vi "FGV Read-write settings-to-Miyachi.vi"(9 "VISA resource name":refnum<visa-resource-name>="COM1", 10 "Soldadora":i32=1, 11 "Linea":i32=1) -> (3 "STATUS":u32(colorbox))   [LabVIEW 2014]
uses:
  control/FGV Variables State machine.ctl
  control/FGV Machine states.ctl
  control/FGV Comandos.ctl
  control/FGV Escribir datos a miyachi-booleano.ctl
  control/FGV Lectura.ctl
  control/FGV botones Read-Write.ctl
  control/FGV Select case.ctl
panel:
  out "current time":timestamp
  in  "min/seg 2":u16(ring) items=["seg", "min"]
  in  "Time update":i32=5
  in  "Exit":bool
  in  "Botones r-w":T1
  out "CURRENT #2":dbl
  out "CURRENT #1":dbl
  out "VOLTLOW2":dbl
  out "VOLTHIW2":dbl
  out "VOLTLOW1":dbl
  out "VOLTHIW1":dbl
  out "Weld mode":i32
  out "Start value":i32
  out "sold1_error_fromLV":bool
  out "sold1_warning_fromLV":bool
  out "error out":errorcluster
  in  "Variables R-W":T2={"Máquina"=0.0, "Error STA"=0.0, "Contador de veces"=0.0, "Timeout"=0.0, "Tiempo"=0.0, "State"=enum."Start", "error in (no error)"={"status"=FALSE, "code"=0, "source"=""}, "error out"={"status"=FALSE, "code"=0, "source"=""}, "Msg Error"="", "Leer comando"="", "up sol"=0.0, "VISA resource name"="", "Comando a recibir"=enum."ACK", "Comando que sigue"=enum."Ninguno", "Modo escritura"=enum."No", "Modo lectura"=enum."No", "Estado Status"=enum."Start", "Botones r-w"={"5"=FALSE, "4"=FALSE, "3"=FALSE, "2"=FALSE, "1"=FALSE}, "stopVI"=FALSE, "Case"=enum."Nada", "Status?"=FALSE, "Soldadora"=0.0}
  in  "error in (no error)":errorcluster
  out "Panel (Local)":bool
  out "PC (Remote)":bool
  out "Local":bool
  out "Remote":bool
  out "FORCE CHANNEL":dbl
  out "Última vez actualizado":string
  out "FORCE":dbl
  out "IMPULSE":dbl
  out "CURRENT #2":string
  out "CURRENT #1":string
  out "%HEAT 2":u32
  out "%HEAT 1":u32
  out "OFF":dbl
  out "HLD":dbl
  out "DN2":dbl
  out "W2":dbl
  out "UP2":dbl
  out "CO":dbl
  out "DN1":dbl
  out "W1":dbl
  out "UP1":dbl
  out "SQZ":dbl
  out "SQD":dbl
  out "Act. SCHE.":dbl
  out "FIRE =":u32
  out "VOLTLOW2":string
  out "VOLTHIW2":string
  out "LO":string
  out "HI":string
  out "HI":dbl
  out "LO":dbl
  out "Weld mode":string
  out "Start value":string
  out "Weld count limit":dbl
  out "Conduction limit #2":dbl
  out "HI":dbl
  out "Low current #2 %":dbl
  out "High current #2 %":dbl
  out "LO":dbl
  out "HI":dbl
  in  "SCHEDULE SET":T8
  in  "MONITOR SET":T9 {"Weld mode" items=["SPOT", "REPEAT", "SUCCESSIVE", "CHAINING"]; "Start value" items=["MAINTAINED", "PULSED", "LATCHED", "SEAM"]}
  in  "SCHEDULE":i32
  in  "SCHEDULE":u32
  out "OK":bool
  # "WELD ON/OFF"
  # "Programming"
  # "CURR(KA)"
  # "COND"
  # "VOLTS"
  # "FORCE(LBS)"
  # "°"
  # "W1"
  # "%"
  # "V"
  # "V"
  # "%"
  # "°"
  # "%"
  # "%"
  # "W2"
  # "V"
  # "V"
  # "Lbs."
  # "VOLTS"
  # "CURR(KA)"
  # "COND"
  # "FORCE(LBS)"
  # "LO"
  # "HI"
  # "HI"
  # "LO"
  # "HI"
  # "LO"
  # "HI"
  # "°"
  # "%"
  # "V"
  # "V"
  # "%"
  # "°"
  # "%"
  # "%"
  # "V"
  # "V"
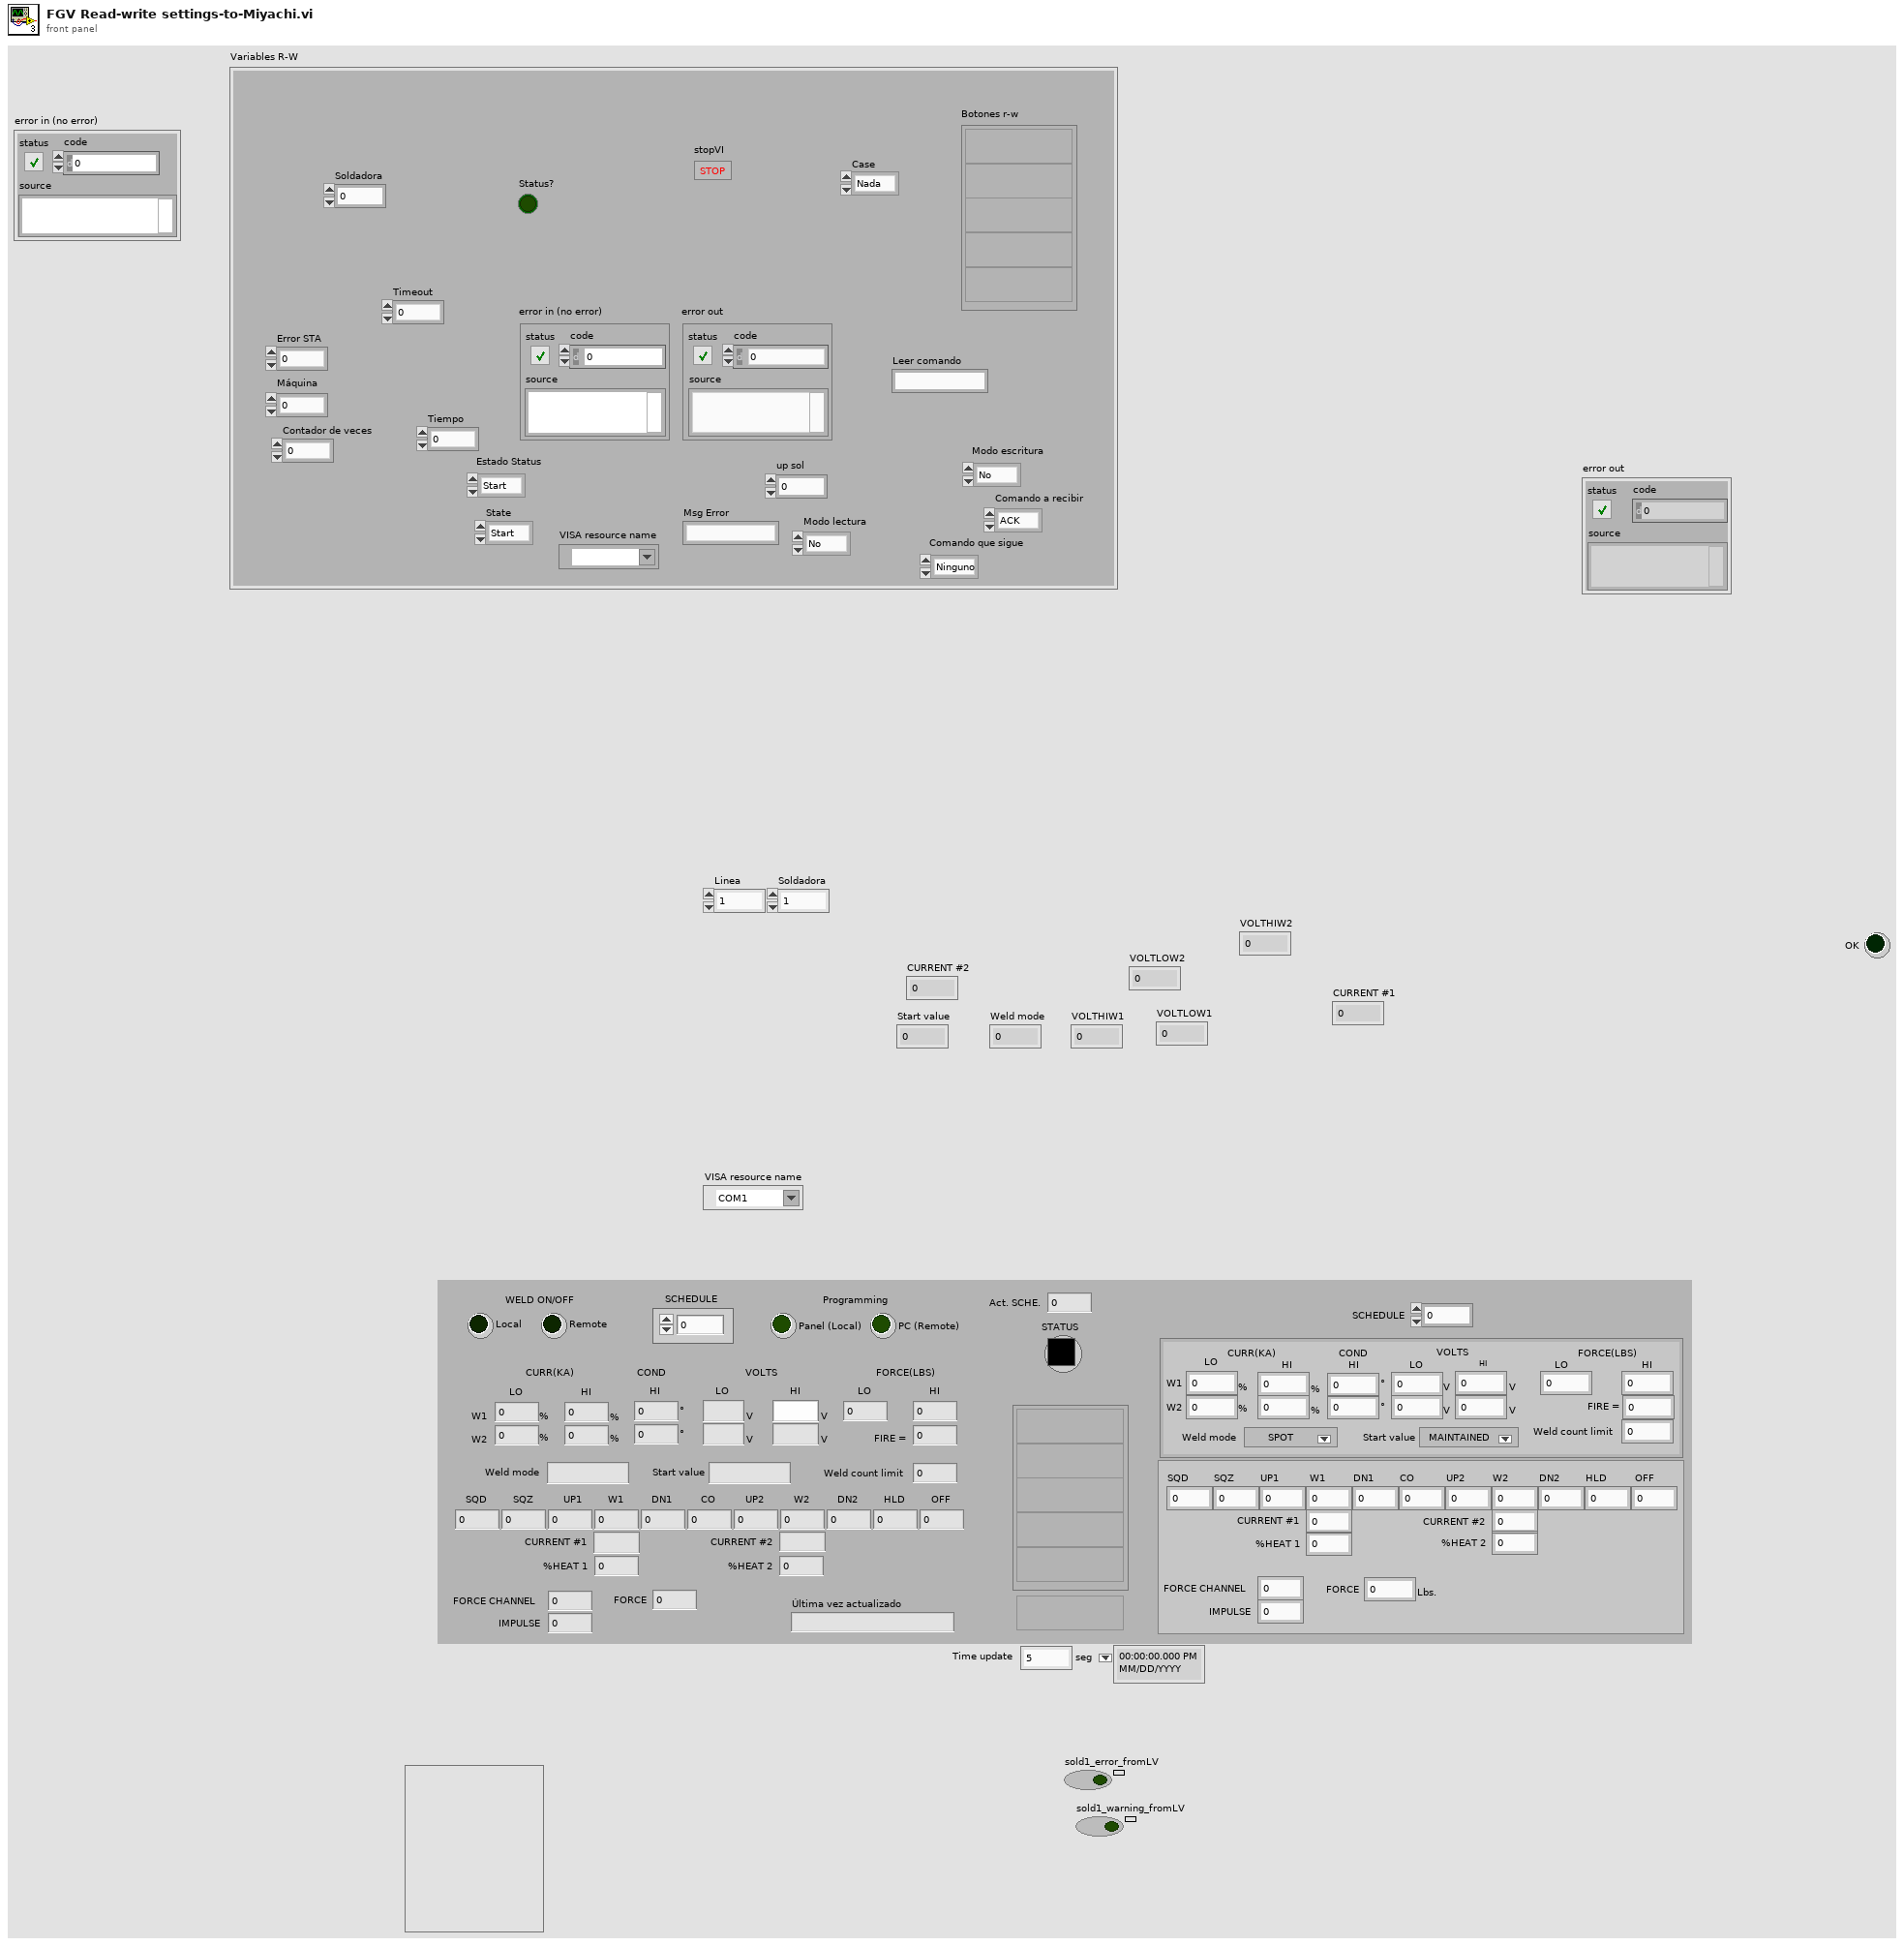
[diagram p1: front panel]
types:
  T1 = typedef "FGV botones Read-Write.ctl" = cluster{"5":bool, "4":bool, "3":bool, "2":bool, "1":bool}
  T2 = typedef "FGV Variables State machine.ctl" = cluster{"Máquina":dbl, "Error STA":dbl, "Contador de veces":dbl, "Timeout":dbl, "Tiempo":dbl, "State":T3, "error in (no error)":errorcluster, "error out":errorcluster, "Msg Error":string, "Leer comando":string, "up sol":dbl, "VISA resource name":refnum<visa-resource-name>, "Comando a recibir":T4, "Comando que sigue":T4, "Modo escritura":T5, "Modo lectura":T6, "Estado Status":T3, "Botones r-w":T1, "stopVI":bool, "Case":T7, "Status?":bool, "Soldadora":dbl}
  T3 = typedef "FGV Machine states.ctl" = enum16{"Start", "Wait", "Send", "Receive", "Error handler", "Show info", "Do something", "Stop", "Idle"}
  T4 = typedef "FGV Comandos.ctl" = enum16{"Ninguno", "ACK", "Monitor Read", "Schedule Read", "Status Read", "Report Read", "Monitor Set", "Schedule Set", "System Read", "Remote", "Load Read", "Load Set", "Reset"}
  T5 = typedef "FGV Escribir datos a miyachi-booleano.ctl" = enum16{"No", "Si"}
  T6 = typedef "FGV Lectura.ctl" = enum16{"No", "Si"}
  T7 = typedef "FGV Select case.ctl" = enum16{"Nada", "Leer", "Escribir", "Local", "Remote", "Activar Sch."}
  T8 = cluster{"SQD":dbl, "SQZ":dbl, "UP1":dbl, " W1":dbl, "DN1":dbl, "CO":dbl, "UP2":dbl, "W2":dbl, "DN2":dbl, "HLD":dbl, " OFF":dbl, "%HEAT 1":dbl, "%HEAT 2":dbl, "CURRENT #1":dbl, " CURRENT #2":dbl, "IMPULSE":dbl, "FORCE":dbl, "FORCE CHANNEL":dbl}
  T9 = cluster{"HIGH1C":u32, " W1":u32, "HIGH2C":u32, "W2":u32, "ANGLE 1":u32, "ANGLE 2":u32, "Weld count limit":u32, "Start value":u16, "Weld mode":u16, "LOP":dbl, "HIP":dbl, "VOLTHIW1":dbl, "VOLTLOW1":dbl, "VOLTHIW2":dbl, "VOLTLOW2":dbl, "FIRE =":dbl}
  T10 = enum16{"Start", "Wait", "Send", "Receive", "Error handler", "Show info", "Do something", "Stop"}
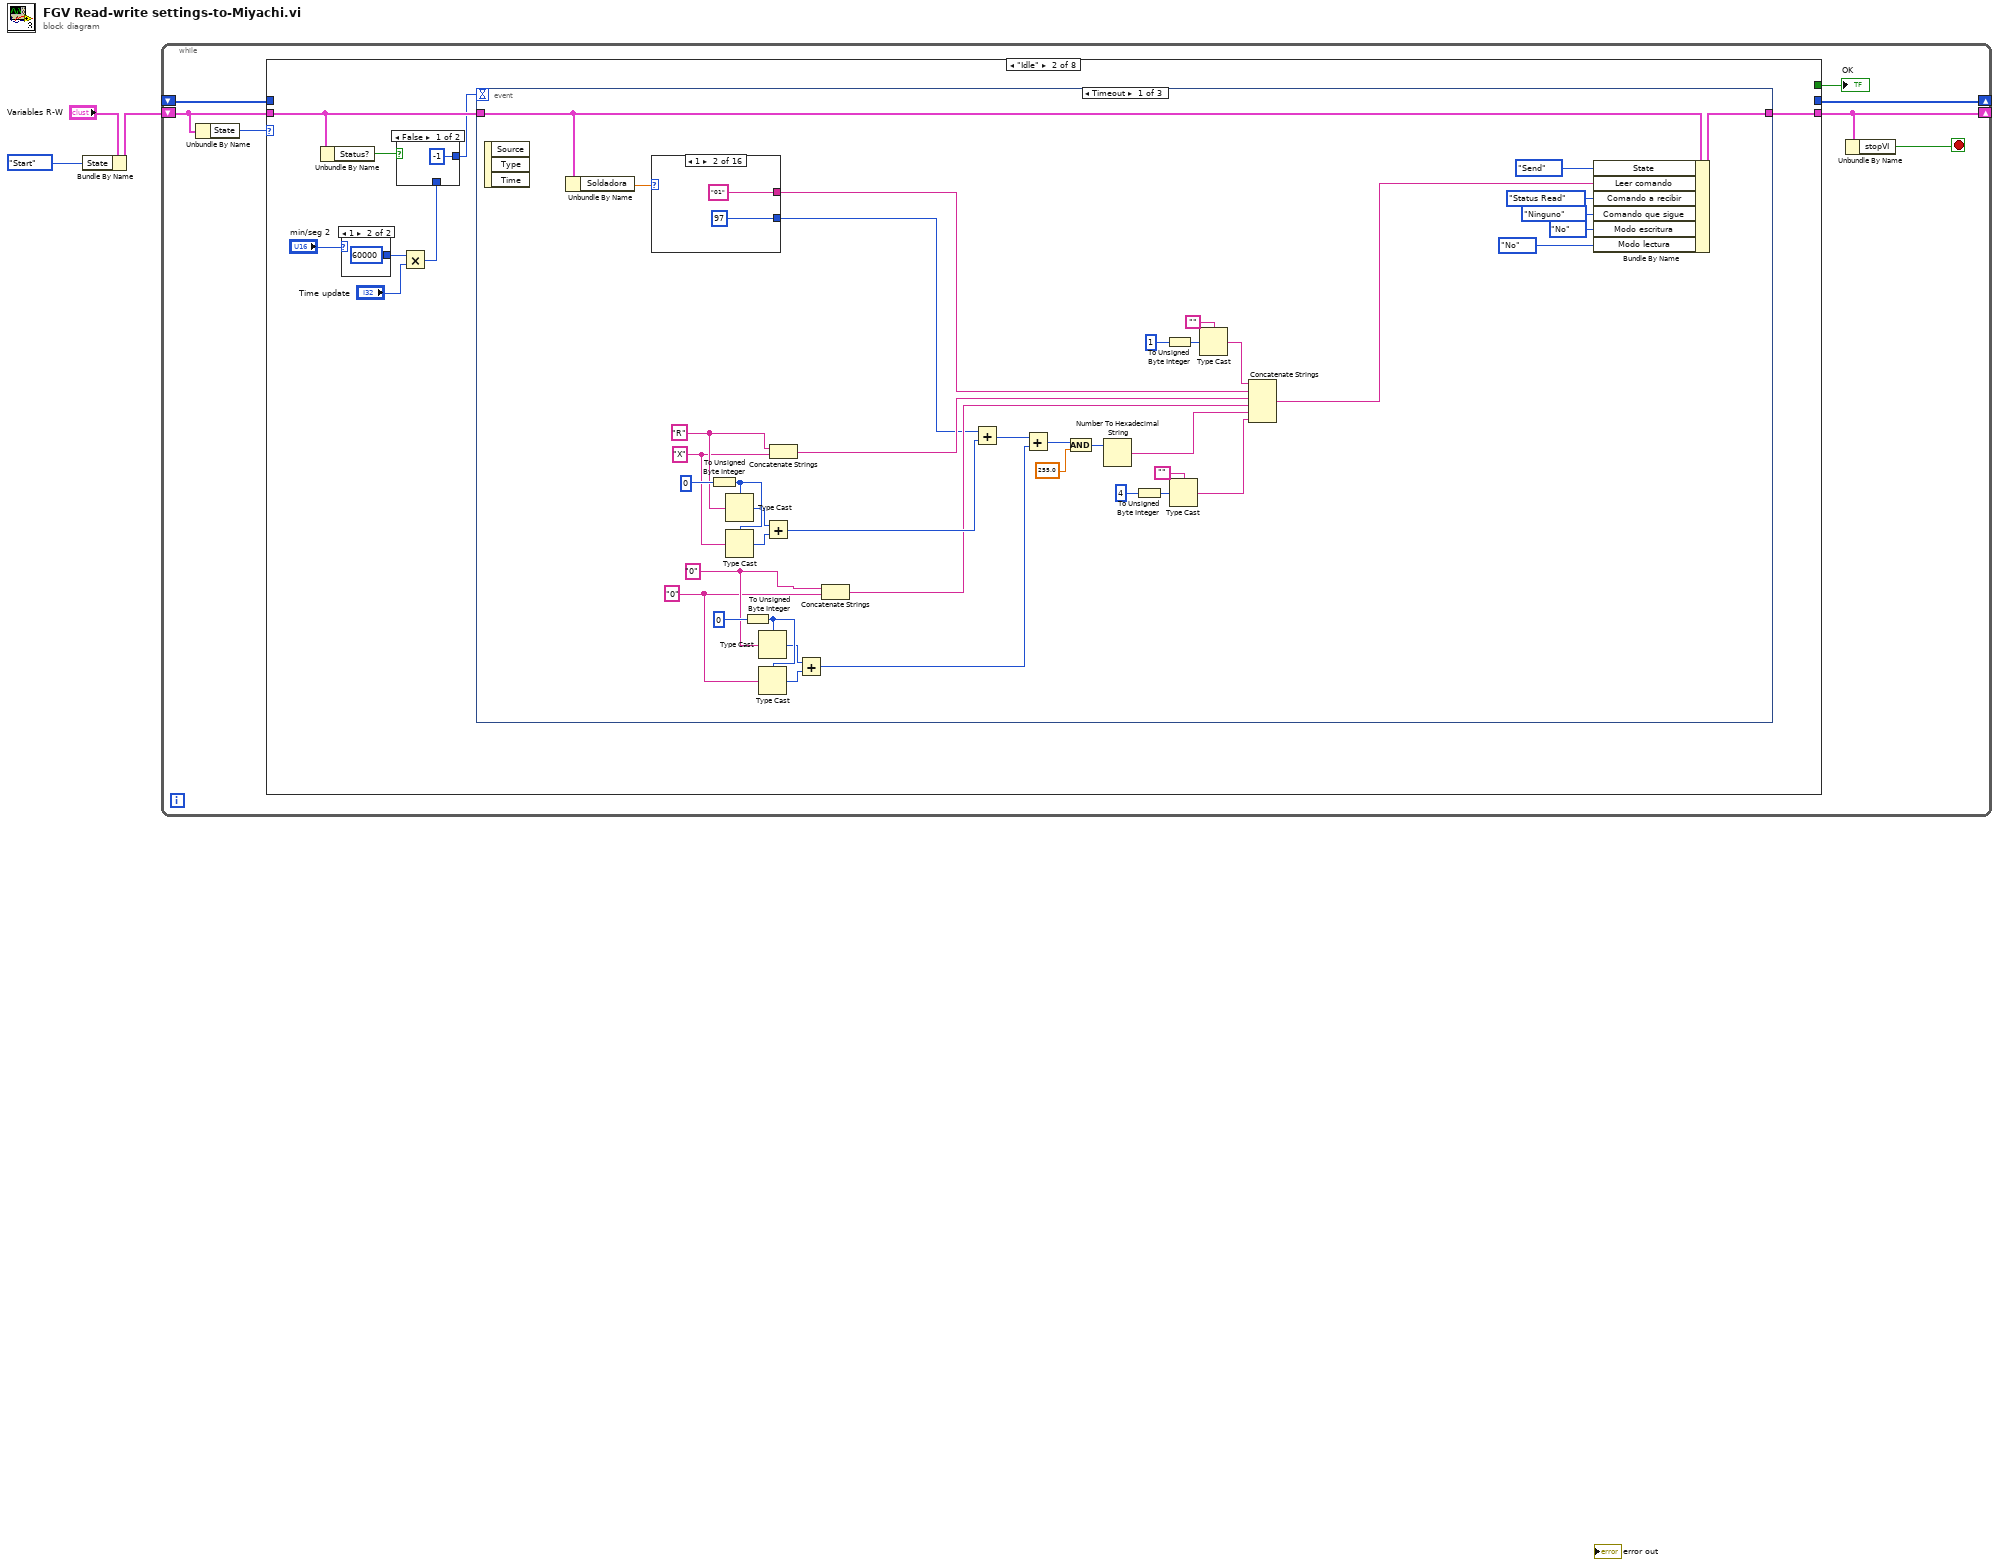
[diagram p0: block diagram]
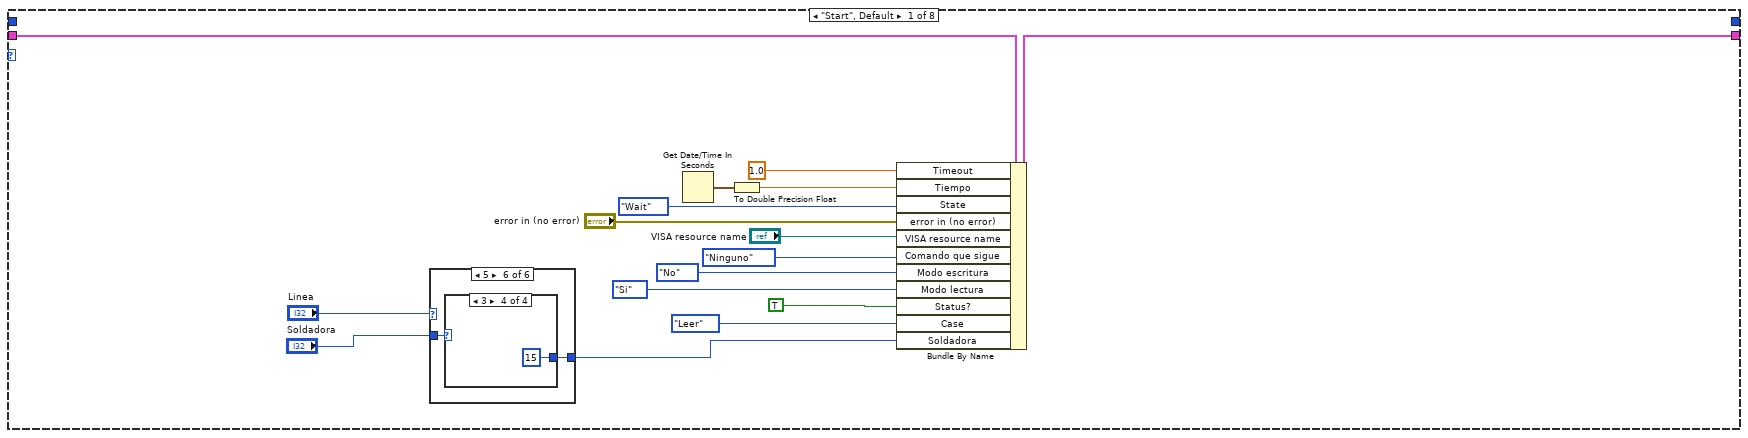
[diagram p2: hidden frame]
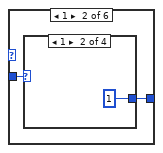
[diagram p4: hidden frame]
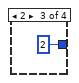
[diagram p6: hidden frame]
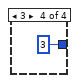
[diagram p7: hidden frame]
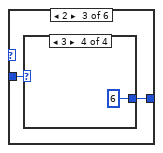
[diagram p8: hidden frame]
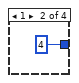
[diagram p10: hidden frame]
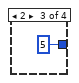
[diagram p11: hidden frame]
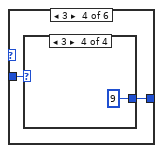
[diagram p12: hidden frame]
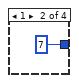
[diagram p14: hidden frame]
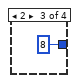
[diagram p15: hidden frame]
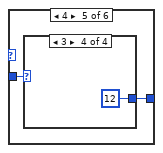
[diagram p16: hidden frame]
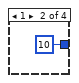
[diagram p18: hidden frame]
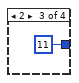
[diagram p19: hidden frame]
diagram:
  n1 = Bundle By Name(cluster="Variables R-W", "State"=FGV_Machine_states."Start" ("Estado R-W")) -> (w1:T2)
  n2 = while {
    shift-right: [w10] -> _
    shift-left: _ -> [w9]
    shift-right: [w5] -> _
    shift-left: w1 -> [w8]
    stop <- w4 stop-if-true
    n3 = Unbundle By Name(w8) -> ("State"=w7:T3)
    n4 = case shown="\"Idle\"" w7 {
      tunnel: [_ _ w192 w523 w537 w597 w747 _] -> w10
      tunnel: w9 -> [_ _ w192 w523 _ w597 w747 _]
      tunnel: [_ _ TRUE FALSE FALSE FALSE FALSE _] -> w6
      tunnel: [w17 w59 w190 w521 w535 w593 w745 w1945] -> w5
      tunnel: w8 -> [w18 w55 w189 w520 w530 w591 w746 w1946]
      frame "Start", Default {
        n5 = case shown="5" "Linea" {
          tunnel: "Soldadora" -> [_ w28 w33 w38 w43 w48]
          tunnel: [_ w27 w32 w37 w42 w47] -> w14
          frame 0, Default {
          }
          frame 1 {
            n6 = case shown="1" w28 {
              tunnel: [_ 1 2 3] -> w27
              frame 0, Default {
              }
              frame 1 {
              }
              frame 2 {
              }
              frame 3 {
              }
            }
          }
          frame 2 {
            n7 = case shown="3" w33 {
              tunnel: [_ 4 5 6] -> w32
              frame 0, Default {
              }
              frame 1 {
              }
              frame 2 {
              }
              frame 3 {
              }
            }
          }
          frame 3 {
            n8 = case shown="3" w38 {
              tunnel: [_ 7 8 9] -> w37
              frame 0, Default {
              }
              frame 1 {
              }
              frame 2 {
              }
              frame 3 {
              }
            }
          }
          frame 4 {
            n9 = case shown="3" w43 {
              tunnel: [_ 10 11 12] -> w42
              frame 0, Default {
              }
              frame 1 {
              }
              frame 2 {
              }
              frame 3 {
              }
            }
          }
          frame 5 {
            n10 = case shown="3" w48 {
              tunnel: [_ 13 14 15] -> w47
              frame 0, Default {
              }
              frame 1 {
              }
              frame 2 {
              }
              frame 3 {
              }
            }
          }
        }
        n11 = Get Date/Time In Seconds() -> (seconds since 1Jan1904=w19:timestamp)
        n12 = To Double Precision Float(number=w19) -> (double precision float=w20:dbl)
        n13 = Bundle By Name(cluster=w18, "Timeout"=1.0, "Tiempo"=w20, "State"=FGV_Machine_states."Wait" ("Estado"), "error in (no error)"="error in (no error)", "VISA resource name"="VISA resource name", "Comando que sigue"=FGV_Comandos."Ninguno" ("Comando en turno"), "Modo escritura"=FGV_Escribir_datos_a_miyachi-booleano."No" ("Escritura?"), "Modo lectura"=FGV_Lectura."Si" ("Lectura"), "Status?"=TRUE, "Case"=FGV_Select_case."Leer", "Soldadora"=w14) -> (w17:T2)
      }
      frame "Idle" {
        n14 = Unbundle By Name(w55) -> ("Status?"=w52:bool)
        n15 = case shown="1" "min/seg 2" {
          tunnel: [1000 60000] -> w58
          frame 0, Default {
          }
          frame 1 {
          }
        }
        n16 = Multiply(x=w58, y="Time update") -> (x*y=w54:i32)
        n17 = case shown="False" w52 {
          tunnel: w54 -> [_ w61]
          tunnel: [-1 w61] -> w53
          frame False {
          }
          frame True {
          }
        }
        n18 = event shown="[0] Timeout" {
          selector: _ -> [_ _ _]
          dyn-events: _ -> [_ _ _]
          timeout: w53 -> [_ _ _]
          tunnel: [w74 w142 w176] -> w59
          tunnel: w55 -> [w71 w136 w177]
          event Timeout {
            w83 = "0" ("string")
            w84 = "0" ("string")
            w95 = "X" ("string")
            w96 = "R" ("string")
            n19 = event-data() -> ()  [unwired: 1 in, 3 out]
            n20 = Unbundle By Name(w71) -> ("Soldadora"=w70:dbl)
            n21 = case shown="1" w70 {
              tunnel: [_ "01" "02" "03" "04" "05" "06" "07" "08" "09" "10" "11" "12" "13" "14" "15"] -> w69
              tunnel: [_ 97 98 99 100 101 102 103 104 105 97 98 99 100 101 102] -> w68
              frame 0, Default {
              }
              frame 1 {
              }
              frame 2 {
              }
              frame 3 {
              }
              frame 4 {
              }
              frame 5 {
              }
              frame 6 {
              }
              frame 7 {
              }
              frame 8 {
              }
              frame 9 {
              }
              frame 10 {
              }
              frame 11 {
              }
              frame 12 {
              }
              frame 13 {
              }
              frame 14 {
              }
              frame 15 {
              }
            }
            n22 = To Unsigned Byte Integer(number=0) -> (unsigned 8bit integer=w99:u8)
            n23 = Type Cast(type=w99, x=w96) -> (*(type *) &x=w98:u8)
            n24 = Type Cast(type=w99, x=w95) -> (*(type *) &x=w97:u8)
            n25 = To Unsigned Byte Integer(number=0) -> (unsigned 8bit integer=w87:u8)
            n26 = Type Cast(type=w87, x=w84) -> (*(type *) &x=w86:u8)
            n27 = Type Cast(type=w87, x=w83) -> (*(type *) &x=w85:u8)
            n28 = Add(x=w98, y=w97) -> (x+y=w91:u8)
            n29 = Concatenate Strings(w96, w95) -> (w79:string)
            n30 = Add(x=w86, y=w85) -> (x+y=w81:u8)
            n31 = Concatenate Strings(w84, w83) -> (w78:string)
            n32 = Add(x=w68, y=w91) -> (x+y=w72:i32)
            n33 = Add(x=w72, y=w81) -> (x+y=w82:i32)
            n34 = And(x=w82, y=255.0) -> (x .and. y?=w89:i32)
            n35 = Number To Hexadecimal String(2:w89) -> (0:w77:string)  [unwired: 1 in]
            n36 = To Unsigned Byte Integer(number=u8 4) -> (unsigned 8bit integer=w94:u8)
            n37 = To Unsigned Byte Integer(number=u8 1) -> (unsigned 8bit integer=w103:u8)
            n38 = Type Cast(type="", x=w94) -> (*(type *) &x=w76:string)
            n39 = Type Cast(type="", x=w103) -> (*(type *) &x=w80:string)
            n40 = Concatenate Strings(w80, w69, w79, w78, w77, w76) -> (w73:string)
            n41 = Bundle By Name(cluster=w71, "State"=FGV_Machine_states."Send" ("Estado R-W"), "Leer comando"=w73, "Comando a recibir"=FGV_Comandos."Status Read", "Comando que sigue"=FGV_Comandos."Ninguno", "Modo escritura"=FGV_Escribir_datos_a_miyachi-booleano."No", "Modo lectura"=FGV_Lectura."No") -> (w74:T2)
          }
          event Value Change {
            n42 = event-data() -> ("CtlRef"=w134:refnum<vi>)  [unwired: 1 in]
            n43 = Cluster To Array(cluster="Botones r-w") -> (array=w148:bool[])
            n44 = for {
              tunnel: w148 -> [w175] mode=indexing
              tunnel: [w174] -> w146
              i -> [w174]
              stop <- w175 stop-if-true
            }
            n45 = property class="Clust"(reference=w134) -> ("Controls[]"=w147:refnum<vi>[])  [unwired: 1 in, 2 out]
            n46 = Index Array(array=w147, index=w146) -> (element=w145:refnum<vi>)
            n47 = Unbundle By Name(w136) -> ("Status?"=w135:bool)
            n48 = property class="Ctl"(reference=w145) -> ("Label.Text"=w144:string)  [unwired: 1 in, 2 out]
            n49 = Decimal String To Number(string=w144) -> (number=w143:i32)  [unwired: 2 in, 1 out]
            n50 = case shown="3" w143 {
              tunnel: [FGV_Machine_states."Idle" ("Estado R-W") FGV_Machine_states."Wait" ("Estado R-W") FGV_Machine_states."Wait" ("Estado R-W") FGV_Machine_states."Wait" ("Estado R-W") FGV_Machine_states."Wait" ("Estado R-W") FGV_Machine_states."Idle" ("Estado R-W")] -> w141
              tunnel: [_ FGV_Lectura."Si" ("Modo lectura") FGV_Lectura."No" ("Modo lectura") FGV_Lectura."No" ("Modo lectura") FGV_Lectura."No" ("Modo lectura") _] -> w140
              tunnel: [_ FGV_Escribir_datos_a_miyachi-booleano."No" ("Modo escritura") FGV_Escribir_datos_a_miyachi-booleano."Si" ("Modo escritura") FGV_Escribir_datos_a_miyachi-booleano."No" ("Modo escritura") FGV_Escribir_datos_a_miyachi-booleano."No" ("Modo escritura") _] -> w139
              tunnel: [_ FGV_Select_case."Leer" ("Case") FGV_Select_case."Escribir" ("Case") FGV_Select_case."Local" ("Case") FGV_Select_case."Remote" ("Case") _] -> w138
              tunnel: [w150 w152 w157 w162 w167 TRUE] -> w137
              tunnel: w135 -> [w150 w152 w157 w162 w167 _]
              frame 0, Default {
              }
              frame 1 {
              }
              frame 2 {
              }
              frame 3 {
              }
              frame 4 {
              }
              frame 5 {
              }
            }
            n51 = Bundle By Name(cluster=w136, "State"=w141, "Modo lectura"=w140, "Modo escritura"=w139, "Case"=w138, "Status?"=w137) -> (w142:T2)
          }
          event "Exit": Value Change {
            n52 = event-data() -> ()  [unwired: 1 in, 6 out]
            n53 = Bundle By Name(cluster=w177, "stopVI"=TRUE) -> (w176:T2)
          }
        }
      }
      frame "Wait" {
        n54 = Unbundle By Name(w189) -> ("Comando que sigue"=w187:T4, "Case"=w180:T7, "Soldadora"=w179:dbl)
        n55 = case shown="\"Escribir\"" w180 {
          tunnel: ["" w220 w297 "\u000101RM01\u000061\u0004" "\u000101RM01\u000162\u0004" "\u000101LS01\u000061\u0004"] -> w188
          tunnel: w187 -> [_ w204 w311 _ _ _]
          tunnel: [w196 w212 w310 FGV_Comandos."Remote" ("Enviar tipo comando") FGV_Comandos."Remote" ("Enviar tipo comando") FGV_Comandos."Load Read" ("Enviar tipo comando")] -> w182
          tunnel: [w196 w211 w309 FGV_Comandos."Ninguno" ("Enviar tipo comando") FGV_Comandos."Ninguno" ("Enviar tipo comando") FGV_Comandos."Ninguno" ("Enviar tipo comando")] -> w183
          tunnel: [FGV_Escribir_datos_a_miyachi-booleano."No" ("Escritura?") FGV_Escribir_datos_a_miyachi-booleano."No" ("Escritura?") w308 FGV_Escribir_datos_a_miyachi-booleano."No" ("Escritura?") FGV_Escribir_datos_a_miyachi-booleano."No" ("Escritura?") FGV_Escribir_datos_a_miyachi-booleano."No" ("Escritura?")] -> w186
          tunnel: [FGV_Lectura."No" ("Lectura") w202 w295 FGV_Lectura."Si" ("Lectura") FGV_Lectura."Si" ("Lectura") FGV_Lectura."No" ("Lectura")] -> w184
          tunnel: "SCHEDULE" -> [_ _ w298 _ _ _]
          tunnel: [FGV_Machine_states."Idle" ("Estado R-W") FGV_Machine_states."Send" ("Estado R-W") FGV_Machine_states."Send" ("Estado R-W") FGV_Machine_states."Send" ("Estado R-W") FGV_Machine_states."Send" ("Estado R-W") FGV_Machine_states."Send" ("Estado R-W")] -> w181
          tunnel: w179 -> [_ w200 w293 _ _ _]
          frame "Nada", Default {
            w196 = FGV_Comandos."Ninguno" ("Enviar tipo comando")
            # "Nada"
          }
          frame "Leer" {
            # "eot"
            # "cksum"
            # "cnt = \"01\"\n'0' + '1' = 97"
            # "Comando"
            # "Máquina"
            # "Monitor read and schedule read"
            n56 = case shown="0, Default" w200 {
              tunnel: [_ "01" "02" "03" "04" "05" "06" "07" "08" "09" "10" "11" "12" "13" "14" "15"] -> w199
              tunnel: [_ 97 98 99 100 101 102 103 104 105 97 98 99 100 101 102] -> w198
              frame 0, Default {
              }
              frame 1 {
              }
              frame 2 {
              }
              frame 3 {
              }
              frame 4 {
              }
              frame 5 {
              }
              frame 6 {
              }
              frame 7 {
              }
              frame 8 {
              }
              frame 9 {
              }
              frame 10 {
              }
              frame 11 {
              }
              frame 12 {
              }
              frame 13 {
              }
              frame 14 {
              }
              frame 15 {
              }
            }
            n57 = case shown="\"Ninguno\", Default" w204 {
              tunnel: ["00" ("string") "00" ("string") "01" ("string")] -> w224
              tunnel: [w257 w263 w269] -> w223
              tunnel: [w257 w263 w267] -> w213
              tunnel: [0 ("SCHEDULE") 0 ("SCHEDULE") "SCHEDULE"] -> w207
              tunnel: [96 ("x") 96 ("x") 97 ("x")] -> w203
              frame "System Read" {
                w257 = ""
              }
              frame "Load Read" {
                w263 = ""
              }
              frame "Ninguno", Default {
                w267 = ""
                # "cnt"
                n58 = To Unsigned Byte Integer(number="SCHEDULE") -> (unsigned 8bit integer=w268:u8)
                n59 = Type Cast(type=w267, x=w268) -> (*(type *) &x=w269:string)
              }
            }
            n60 = To Unsigned Byte Integer(number=4) -> (unsigned 8bit integer=w217:u8)
            n61 = Type Cast(type=w213, x=w217) -> (*(type *) &x=w221:string)
            n62 = case shown="\"Load Read\"" w204 {
              tunnel: ["MR" "DR" "YR" "LR"] -> w215
              tunnel: [159 150 171 158] -> w209
              frame "Monitor Read", Default {
              }
              frame "Schedule Read" {
              }
              frame "System Read" {
              }
              frame "Load Read" {
              }
            }
            n63 = Add(x=w198, y=w209) -> (x+y=w208:i32)
            n64 = Add(x=w208, y=w207) -> (x+y=w205:i32)
            n65 = Add(x=w203, y=w205) -> (x+y=w206:i32)
            n66 = To Unsigned Byte Integer(number=w206) -> (unsigned 8bit integer=w214:u8)
            n67 = Number To Hexadecimal String(2:w214) -> (0:w222:string)  [unwired: 1 in]
            n68 = To Unsigned Byte Integer(number=1) -> (unsigned 8bit integer=w219:u8)
            n69 = Type Cast(type="", x=w219) -> (*(type *) &x=w225:string)
            n70 = case shown="\"Schedule Read\"" w204 {
              tunnel: [FGV_Comandos."Monitor Read" ("Enviar tipo comando") FGV_Comandos."Schedule Read" ("Enviar tipo comando") FGV_Comandos."System Read" ("Enviar tipo comando") FGV_Comandos."Load Read" ("Enviar tipo comando")] -> w212
              tunnel: [FGV_Comandos."Schedule Read" ("Comando en turno") FGV_Comandos."System Read" ("Comando en turno") FGV_Comandos."Load Read" ("Comando en turno") FGV_Comandos."Ninguno" ("Comando en turno")] -> w211
              tunnel: [FGV_Lectura."Si" ("Lectura") FGV_Lectura."Si" ("Lectura") FGV_Lectura."Si" ("Lectura") FGV_Lectura."No" ("Lectura")] -> w202
              frame "Monitor Read", Default {
              }
              frame "Schedule Read" {
              }
              frame "System Read" {
              }
              frame "Load Read" {
              }
            }
            n71 = Concatenate Strings(w225, w199, w215, w224, w223, w222, w221) -> (w220:string)
          }
          frame "Escribir" {
            # "<soh>\n<@>\n<cmd>\n<cnt>\n<data>\n<cksm>\n<eot>"
            n72 = case shown="0, Default" w293 {
              tunnel: [_ "01" "02" "03" "04" "05" "06" "07" "08" "09" "10" "11" "12" "13" "14" "15"] -> w291
              tunnel: [_ 97 98 99 100 101 102 103 104 105 97 98 99 100 101 102] -> w292
              frame 0, Default {
              }
              frame 1 {
              }
              frame 2 {
              }
              frame 3 {
              }
              frame 4 {
              }
              frame 5 {
              }
              frame 6 {
              }
              frame 7 {
              }
              frame 8 {
              }
              frame 9 {
              }
              frame 10 {
              }
              frame 11 {
              }
              frame 12 {
              }
              frame 13 {
              }
              frame 14 {
              }
              frame 15 {
              }
            }
            n73 = To Unsigned Byte Integer(number=w298) -> (unsigned 8bit integer=w319:u8)
            n74 = Type Cast(type="", x=w319) -> (*(type *) &x=w303:string)
            n75 = case shown="\"Schedule Set\"" w311 {
              tunnel: [w363 w445] -> w302
              tunnel: [w362 w450] -> w300
              tunnel: [FGV_Comandos."Monitor Set" ("Enviar tipo comando") FGV_Comandos."Schedule Set" ("Enviar tipo comando")] -> w310
              tunnel: [FGV_Comandos."Schedule Set" ("Enviar tipo comando") FGV_Comandos."Ninguno" ("Enviar tipo comando")] -> w309
              tunnel: [FGV_Escribir_datos_a_miyachi-booleano."Si" ("Escritura?") FGV_Escribir_datos_a_miyachi-booleano."No" ("Escritura?")] -> w308
              tunnel: [w357 "DS" ("string")] -> w305
              tunnel: [w350 "23" ("string")] -> w304
              tunnel: w303 -> [w364 w446]
              tunnel: w298 -> [w359 w443]
              tunnel: [FGV_Lectura."No" ("Lectura") FGV_Lectura."Si" ("Lectura")] -> w295
              frame "Monitor Set", Default {
                # "MONITOR SET \"MS\""
                n76 = property on="MONITOR SET" class="Clust (strict)"() -> ("Controls[]"=w373:refnum<vi>[])  [unwired: 2 in, 2 out]
                n77 = for {
                  N: 16 -> [_]
                  tunnel: w373 -> [w384] mode=indexing
                  shift-right: [w379] -> w365
                  shift-left: "" -> [w380]
                  shift-right: [w376] -> w366
                  shift-left: 0 -> [w382]
                  i -> [w374]
                  n78 = property class="Ctl"(reference=w384) -> ("Value"=w383:variant)  [unwired: 1 in, 2 out]
                  n79 = Variant To Data(type=0.0 ("y"), Variant=w383) -> (data=w381:dbl)  [unwired: 1 in, 1 out]
                  n80 = case shown="8" w374 {
                    tunnel: w381 -> [w385 w387 w391 w395 w401 w405 w409 w417 w425 w433]
                    tunnel: [w386 w388 w392 w399 w402 w406 w410 w418 w427 w434] -> w378
                    tunnel: [w385 w387 w391 w396 w401 w405 w412 w421 w428 w436] -> w375
                    frame 0, Default {
                      n81 = call "Number-to-two_ASCII_char.vi"("two_byte_num"=w385) -> ("two_ascii_string"=w386:string)  [unwired: 10 in]
                    }
                    frame 4 {
                      n82 = To Unsigned Byte Integer(number=w387) -> (unsigned 8bit integer=w390:u8)
                      n83 = Type Cast(type="", x=w390) -> (*(type *) &x=w388:string)
                    }
                    frame 5 {
                      n84 = To Unsigned Byte Integer(number=w391) -> (unsigned 8bit integer=w394:u8)
                      n85 = Type Cast(type="", x=w394) -> (*(type *) &x=w392:string)
                    }
                    frame 6 {
                      n86 = Quotient & Remainder(x=w395, y=256.0) -> (x-y*floor(x/y)=w398:dbl, floor(x/y)=w397:dbl)
                      n87 = Add(x=w398, y=w397) -> (x+y=w396:dbl)
                      n88 = call "Number-to-two_ASCII_char.vi"("two_byte_num"=w395) -> ("two_ascii_string"=w399:string)  [unwired: 10 in]
                    }
                    frame 7 {
                      n89 = To Unsigned Byte Integer(number=w401) -> (unsigned 8bit integer=w404:u8)
                      n90 = Type Cast(type="", x=w404) -> (*(type *) &x=w402:string)
                    }
                    frame 8 {
                      n91 = To Unsigned Byte Integer(number=w405) -> (unsigned 8bit integer=w408:u8)
                      n92 = Type Cast(type="", x=w408) -> (*(type *) &x=w406:string)
                    }
                    frame 11 {
                      n93 = Multiply(x=w409, y=100.0) -> (x*y=w411:dbl)
                      n94 = Quotient & Remainder(x=w411, y=256.0) -> (x-y*floor(x/y)=w414:dbl, floor(x/y)=w413:dbl)
                      n95 = Add(x=w414, y=w413) -> (x+y=w412:dbl)
                      n96 = call "Number-to-two_ASCII_char.vi"("two_byte_num"=w411) -> ("two_ascii_string"=w410:string)  [unwired: 10 in]
                    }
                    frame 12 {
                      n97 = Multiply(x=w417, y=100.0) -> (x*y=w419:dbl)
                      n98 = Quotient & Remainder(x=w419, y=256.0) -> (x-y*floor(x/y)=w423:dbl, floor(x/y)=w422:dbl)
                      n99 = Add(x=w423, y=w422) -> (x+y=w421:dbl)
                      n100 = call "Number-to-two_ASCII_char.vi"("two_byte_num"=w419) -> ("two_ascii_string"=w418:string)  [unwired: 10 in]
                    }
                    frame 13 {
                      n101 = Multiply(x=w425, y=100.0) -> (x*y=w426:dbl)
                      n102 = Quotient & Remainder(x=w426, y=256.0) -> (x-y*floor(x/y)=w430:dbl, floor(x/y)=w429:dbl)
                      n103 = Add(x=w430, y=w429) -> (x+y=w428:dbl)
                      n104 = call "Number-to-two_ASCII_char.vi"("two_byte_num"=w426) -> ("two_ascii_string"=w427:string)  [unwired: 10 in]
                    }
                    frame 14 {
                      n105 = Multiply(x=w433, y=100.0) -> (x*y=w435:dbl)
                      n106 = Quotient & Remainder(x=w435, y=256.0) -> (x-y*floor(x/y)=w438:dbl, floor(x/y)=w437:dbl)
                      n107 = Add(x=w438, y=w437) -> (x+y=w436:dbl)
                      n108 = call "Number-to-two_ASCII_char.vi"("two_byte_num"=w435) -> ("two_ascii_string"=w434:string)  [unwired: 10 in]
                    }
                  }
                  n109 = Add(x=w382, y=w375) -> (x+y=w376:dbl)
                  n110 = Concatenate Strings(w380, w378) -> (w379:string)
                }
                n111 = call "two-char-cksum.vi"("B"="S" ("string"), "A"="M" ("string")) -> ("CKSUM"=w354:u8, "concatenated string"=w357:string)  [unwired: 8 in]
                n112 = call "two-char-cksum.vi"("B"="D" ("string"), "A"="1" ("string")) -> ("CKSUM"=w351:u8, "concatenated string"=w350:string)  [unwired: 8 in]
                n113 = Add(x=w351, y=w354) -> (x+y=w360:u8)
                n114 = Add(x=w366, y=w359) -> (x+y=w361:dbl)
                n115 = Concatenate Strings(w364, w365) -> (w363:string)
                n116 = Add(x=w361, y=w360) -> (x+y=w362:dbl)
              }
              frame "Schedule Set" {
                # "Escritura de datos de soldadora 1."
                # "SCHEDULE SET \"DS\""
                n117 = property on="SCHEDULE SET" class="Clust (strict)"() -> ("Controls[]"=w458:refnum<vi>[])  [unwired: 2 in, 2 out]
                n118 = for {
                  N: 18 -> [_]
                  tunnel: w458 -> [w464] mode=indexing
                  shift-right: [w459] -> w451
                  shift-left: u8 0 ("number") -> [w465]
                  shift-right: [w467] -> w447
                  shift-left: "" -> [w469]
                  i -> [w466]
                  n119 = property class="Ctl"(reference=w464) -> ("Value"=w463:variant)  [unwired: 1 in, 2 out]
                  n120 = Variant To Data(type=0.0 ("y"), Variant=w463) -> (data=w462:dbl)  [unwired: 1 in, 1 out]
                  n121 = case shown="13" w466 {
                    tunnel: w462 -> [w470 w478 w480 w488 w492]
                    tunnel: [w471 w479 w487 w491 w495] -> w468
                    tunnel: [w470 w473 w482 w488 w492] -> w460
                    frame 0, Default {
                      n122 = call "Number-to-two_ASCII_char.vi"("two_byte_num"=w470) -> ("two_ascii_string"=w471:string)  [unwired: 10 in]
                    }
                    frame 13 {
                      n123 = Multiply(x=w478, y=100.0) -> (x*y=w477:dbl)
                      n124 = Quotient & Remainder(x=w477, y=256.0) -> (x-y*floor(x/y)=w475:dbl, floor(x/y)=w474:dbl)
                      n125 = Add(x=w475, y=w474) -> (x+y=w473:dbl)
                      n126 = call "Number-to-two_ASCII_char.vi"("two_byte_num"=w477) -> ("two_ascii_string"=w479:string)  [unwired: 10 in]
                    }
                    frame 14 {
                      n127 = Multiply(x=w480, y=100.0) -> (x*y=w486:dbl)
                      n128 = Quotient & Remainder(x=w486, y=256.0) -> (x-y*floor(x/y)=w484:dbl, floor(x/y)=w483:dbl)
                      n129 = Add(x=w484, y=w483) -> (x+y=w482:dbl)
                      n130 = call "Number-to-two_ASCII_char.vi"("two_byte_num"=w486) -> ("two_ascii_string"=w487:string)  [unwired: 10 in]
                    }
                    frame 15 {
                      n131 = To Unsigned Byte Integer(number=w488) -> (unsigned 8bit integer=w489:u8)
                      n132 = Type Cast(type="", x=w489) -> (*(type *) &x=w491:string)
                    }
                    frame 17 {
                      n133 = To Unsigned Byte Integer(number=w492) -> (unsigned 8bit integer=w493:u8)
                      n134 = Type Cast(type="", x=w493) -> (*(type *) &x=w495:string)
                    }
                  }
                  n135 = Add(x=w465, y=w460) -> (x+y=w459:dbl)
                  n136 = Concatenate Strings(w469, w468) -> (w467:string)
                }
                n137 = Add(x=w443, y=252.0) -> (x+y=w442:dbl)
                n138 = Add(x=w451, y=w442) -> (x+y=w450:dbl)
                n139 = Concatenate Strings(w446, w447) -> (w445:string)
              }
            }
            n140 = To Unsigned Byte Integer(number=u8 1) -> (unsigned 8bit integer=w318:u8)
            n141 = Add(x=w300, y=w292) -> (x+y=w299:dbl)
            n142 = Type Cast(type="", x=w318) -> (*(type *) &x=w313:string)
            n143 = And(x=w299, y=255.0) -> (x .and. y?=w296:i32)
            n144 = To Unsigned Byte Integer(number=u8 4) -> (unsigned 8bit integer=w314:u8)
            n145 = Number To Hexadecimal String(2:w296) -> (0:w316:string)  [unwired: 1 in]
            n146 = Type Cast(type=w316, x=w314) -> (*(type *) &x=w315:string)
            n147 = Concatenate Strings(w313, w291, w305, w304, w302, w316, w315) -> (w297:string)
          }
          frame "Local" {
            # "Local"
          }
          frame "Remote" {
            # "Programar"
          }
          frame "Activar Sch." {
            # "Set Active Schedule"
          }
        }
        n148 = Bundle By Name(cluster=w189, "State"=w181, "Leer comando"=w188, "Modo lectura"=w184, "Comando que sigue"=w183, "Comando a recibir"=w182, "Modo escritura"=w186) -> (w190:T2)
      }
      frame "Send" {
        n149 = Unbundle By Name(w520) -> ("VISA resource name"=w516:refnum<visa-resource-name>, "Leer comando"=w514:string, "Timeout"=w515:dbl, "error in (no error)"=w517:errorcluster)
        n150 = call "2. FGV Write and read.vi"("error in (no error)"=w517, "Timeout (s)"=w515, "Command"=w514, "VISA resource name"=w516) -> ("error out"=w518:errorcluster)  [unwired: 7 in]
        n151 = Select(t=T10."Error handler" ("Enum"), s=w518, f=T10."Receive" ("Enum")) -> (s? t:f=w519:T10)
        n152 = Bundle By Name(cluster=w520, "State"=w519, "error in (no error)"=w518) -> (w521:T2)
      }
      frame "Receive" {
        n153 = Unbundle By Name(w530) -> ("VISA resource name"=w526:refnum<visa-resource-name>, "error in (no error)"=w527:errorcluster)
        n154 = call "11. FGV Message check.vi"("VISA resource name"=w526, "error in (no error)"=w527) -> ("Err"=w532:i32, "Machine"=w534:i32, "Cmd"=w533:string, "Data"=w537:i32[], "error out"=w529:errorcluster)  [unwired: 8 in, 1 out]
        n155 = case shown="No Error" w529 {
          selector: w529 -> [w541 w584]
          tunnel: w532 -> [w542 _]
          tunnel: [w540 w584] -> w528
          frame No Error {
            n156 = case shown="8" w542 {
              tunnel: w541 -> [w543 w547 w549 w554 w559 w564 w569 w574 w579]
              tunnel: [w543 w546 w550 w555 w560 w565 w570 w575 w580] -> w540
              frame 0, Default {
                # "NO ERROR"
              }
              frame 1 {
                # "NO SOH"
                n157 = Bundle By Name(cluster=w547, "status"=TRUE, "code"=-1, "source"="STA error") -> (w546:errorcluster)
              }
              frame 2 {
                # "BAD CHECKSUM"
                n158 = Bundle By Name(cluster=w549, "status"=TRUE, "code"=-5, "source"="STA error") -> (w550:errorcluster)
              }
              frame 3 {
                # "UNRECOGNIZED COMMAND"
                n159 = Bundle By Name(cluster=w554, "status"=TRUE, "code"=-6, "source"="STA error") -> (w555:errorcluster)
              }
              frame 4 {
                # "TIMEOUT"
                n160 = Bundle By Name(cluster=w559, "status"=TRUE, "code"=2, "source"="STA error") -> (w560:errorcluster)
              }
              frame 5 {
                # "HC16 IS BUSY"
                n161 = Bundle By Name(cluster=w564, "status"=TRUE, "code"=1, "source"="STA error") -> (w565:errorcluster)
              }
              frame 6 {
                # "DATA BAD"
                n162 = Bundle By Name(cluster=w569, "status"=TRUE, "code"=-7, "source"="STA error") -> (w570:errorcluster)
              }
              frame 7 {
                # "INPUT TIMEOUT"
                n163 = Bundle By Name(cluster=w574, "status"=TRUE, "code"=3, "source"="STA error") -> (w575:errorcluster)
              }
              frame 8 {
                # "OUTPUT TIMEOUT"
                n164 = Bundle By Name(cluster=w579, "status"=TRUE, "code"=4, "source"="STA error") -> (w580:errorcluster)
              }
            }
          }
          frame Error {
          }
        }
        n165 = Select(t=T10."Error handler" ("Enum"), s=w528, f=T10."Do something" ("Enum")) -> (s? t:f=w531:T10)
        n166 = Bundle By Name(cluster=w530, "Leer comando"=w533, "Máquina"=w534, "Error STA"=w532, "State"=w531, "error in (no error)"=w528) -> (w535:T2)
      }
      frame "Error handler" {
        n167 = Unbundle By Name(w591) -> ("Timeout"=w595:dbl, "Contador de veces"=w594:dbl, "error in (no error)"=w587:errorcluster)
        n168 = call "10. FGV Error handler.vi"("error in (no error)"=w587) -> ("Error message"=w586:string, "Error code"=w585:i32)  [unwired: 17 in]
        n169 = case shown="-5" w585 {
          tunnel: w595 -> [w599 w601 w616 w627 w642 w653 w669 w686 w693 w696 w702 w715 w729]
          tunnel: w586 -> [_ w608 w621 w634 w641 w658 w668 w684 _ _ w703 w716 w728]
          tunnel: w594 -> [w598 w604 w614 w630 w640 w656 w673 w681 w692 w695 w698 w711 w724]
          tunnel: [T10."Wait" ("Enum") w602 w617 w629 w644 w654 w666 w683 T10."Wait" ("Enum") T10."Wait" ("Enum") w700 w712 w726] -> w592
          tunnel: [w599 w601 w616 w627 w643 w653 w667 w682 w693 w696 w699 w713 w725] -> w590
          tunnel: [w598 w603 w615 w628 w640 w655 w673 w681 w692 w695 w698 w711 w724] -> w589
          frame -1073807360 {
            # "Descripción: Checar si la tarjeta de comunicación no ha sido desconectada."
            # "Unknown system error (miscellaneous error)."
          }
          frame -7 {
            # "Data bad"
            n170 = Increment(x=w604) -> (x+1=w605:dbl)
            n171 = Less?(x=5, y=w605) -> (x < y?=w606:bool)
            n172 = case shown="True" w606 {
              tunnel: w608 -> [_ w613]
              tunnel: w605 -> [w610 _]
              tunnel: [w610 0] -> w603
              tunnel: [T10."Send" ("Enum") T10."Wait" ("Enum")] -> w602
              frame False {
              }
              frame True {
                n173 = call "Display Message to User"("Message"=w613) -> ()  [unwired: 9 in, 2 out]
              }
            }
          }
          frame -6 {
            # "Unrecognized command"
            n174 = Increment(x=w614) -> (x+1=w618:dbl)
            n175 = Less?(x=5, y=w618) -> (x < y?=w619:bool)
            n176 = case shown="True" w619 {
              tunnel: w621 -> [_ w626]
              tunnel: w618 -> [w623 _]
              tunnel: [w623 0] -> w615
              tunnel: [T10."Send" ("Enum") T10."Wait" ("Enum")] -> w617
              frame False {
              }
              frame True {
                n177 = call "Display Message to User2"("Message"=w626) -> ()  [unwired: 9 in, 2 out]
              }
            }
          }
          frame -5 {
            # "Bad Checksum"
            n178 = Increment(x=w630) -> (x+1=w631:dbl)
            n179 = Less?(x=3, y=w631) -> (x < y?=w632:bool)
            n180 = case shown="True" w632 {
              tunnel: w634 -> [_ w639]
              tunnel: w631 -> [w636 _]
              tunnel: [w636 0] -> w628
              tunnel: [T10."Send" ("Enum") T10."Wait" ("Enum")] -> w629
              frame False {
              }
              frame True {
                n181 = call "Display Message to User3"("Message"=w639) -> ()  [unwired: 9 in, 2 out]
              }
            }
          }
          frame -4 {
            n182 = Increment(x=w642) -> (x+1=w645:dbl)
            n183 = Less?(x=4.0 ("y"), y=w645) -> (x < y?=w647:bool)
            n184 = case shown="True" w647 {
              tunnel: w645 -> [w649 _]
              tunnel: [w649 1.0] -> w643
              tunnel: w641 -> [_ w651]
              tunnel: [T10."Send" ("Enum") T10."Wait" ("Enum")] -> w644
              frame False {
              }
              frame True {
                n185 = call "Display Message to User4"("Message"=w651) -> ()  [unwired: 9 in, 2 out]
              }
            }
          }
          frame -3 {
            # "Bad counter"
            n186 = Increment(x=w656) -> (x+1=w657:dbl)
            n187 = Less?(x=5, y=w657) -> (x < y?=w659:bool)
            n188 = case shown="True" w659 {
              tunnel: w658 -> [_ w665]
              tunnel: w657 -> [w662 _]
              tunnel: [w662 0] -> w655
              tunnel: [T10."Send" ("Enum") T10."Wait" ("Enum")] -> w654
              frame False {
              }
              frame True {
                n189 = call "Display Message to User5"("Message"=w665) -> ()  [unwired: 9 in, 2 out]
              }
            }
          }
          frame -2 {
            # "Timeout: Empty buffer"
            n190 = Increment(x=w669) -> (x+1=w670:dbl)
            n191 = Less?(x=4.0 ("y"), y=w670) -> (x < y?=w672:bool)
            n192 = case shown="True" w672 {
              tunnel: w670 -> [w675 _]
              tunnel: [w675 1.0] -> w667
              tunnel: w668 -> [_ w677]
              tunnel: [T10."Send" ("Enum") T10."Wait" ("Enum")] -> w666
              frame False {
              }
              frame True {
                n193 = call "Display Message to User6"("Message"=w677) -> ()  [unwired: 9 in, 2 out]
              }
            }
          }
          frame -1 {
            # "Incrementa timeout"
            # "Timeout: SOH not found"
            n194 = Increment(x=w686) -> (x+1=w679:dbl)
            n195 = Less?(x=4.0 ("y"), y=w679) -> (x < y?=w685:bool)
            n196 = case shown="True" w685 {
              tunnel: w679 -> [w688 _]
              tunnel: [w688 1.0] -> w682
              tunnel: w684 -> [_ w690]
              tunnel: [T10."Send" ("Enum") T10."Wait" ("Enum")] -> w683
              frame False {
              }
              frame True {
                n197 = call "Display Message to User7"("Message"=w690) -> ()  [unwired: 9 in, 2 out]
              }
            }
          }
          frame 0, Default {
          }
          frame 1 {
            # "HC16 IS BUSY"
          }
          frame 2 {
            # "Incrementa timeout"
            # "TIMEOUT STA"
            n198 = Increment(x=w702) -> (x+1=w705:dbl)
            n199 = Greater Or Equal?(x=w705, y=4.0) -> (x >= y?=w704:bool)
            n200 = case shown="True" w704 {
              tunnel: w705 -> [w707 _]
              tunnel: [w707 1.0] -> w699
              tunnel: w703 -> [_ w709]
              tunnel: [T10."Send" ("Enum") T10."Wait" ("Enum")] -> w700
              frame False {
              }
              frame True {
                n201 = call "Display Message to User8"("Message"=w709) -> ()  [unwired: 9 in, 2 out]
              }
            }
          }
          frame 3 {
            # "Incrementa timeout"
            # "INPUT TIMEOUT STA"
            n202 = Increment(x=w715) -> (x+1=w718:dbl)
            n203 = Greater Or Equal?(x=w718, y=4.0) -> (x >= y?=w717:bool)
            n204 = case shown="True" w717 {
              tunnel: w718 -> [w720 _]
              tunnel: [w720 1.0] -> w713
              tunnel: w716 -> [_ w722]
              tunnel: [T10."Send" ("Enum") T10."Wait" ("Enum")] -> w712
              frame False {
              }
              frame True {
                n205 = call "Display Message to User9"("Message"=w722) -> ()  [unwired: 9 in, 2 out]
              }
            }
          }
          frame 4 {
            # "Incrementa timeout"
            # "OUTPUT TIMEOUT STA"
            n206 = Increment(x=w729) -> (x+1=w731:dbl)
            n207 = Greater Or Equal?(x=w731, y=4.0) -> (x >= y?=w730:bool)
            n208 = case shown="True" w730 {
              tunnel: w731 -> [w733 _]
              tunnel: [w733 1.0] -> w725
              tunnel: w728 -> [_ w735]
              tunnel: [T10."Send" ("Enum") T10."Wait" ("Enum")] -> w726
              frame False {
              }
              frame True {
                n209 = call "Display Message to User10"("Message"=w735) -> ()  [unwired: 9 in, 2 out]
              }
            }
          }
        }
        n210 = Bundle By Name(cluster=w591, "State"=w592, "Timeout"=w590, "Contador de veces"=w589, "error in (no error).status"=FALSE, "Msg Error"=w586) -> (w593:T2)
      }
      frame "Do something" {
        n211 = Unbundle By Name(w746) -> ("Modo lectura"=w741:T6, "Modo escritura"=w742:T5, "Comando a recibir"=w743:T4, "Case"=w737:T7)
        n212 = case shown="\"Schedule Read\"" w743 {
          tunnel: w747 -> [_ w756 w899 w903 w1047 w1233 w1348 _ _ _ _]
          tunnel: [TRUE TRUE TRUE TRUE w1040 TRUE TRUE TRUE TRUE TRUE TRUE] -> w739
          tunnel: [w751 w753 w895 w900 w1038 w1192 w1345 w1715 w1717 w1940 FGV_Select_case."Leer" ("Case")] -> w738
          tunnel: w737 -> [w751 w753 w895 w900 w1038 w1192 w1345 w1715 w1717 w1940 _]
          frame "Ninguno", Default {
          }
          frame "Monitor Read" {
            n213 = for {
              N: 29 -> [_]
              shift-right: [w763] -> _
              shift-left: w756 -> [w759]
              shift-right: [w762] -> _
              shift-left: "" -> [w761]
              i -> [w760]
              n214 = Index Array(array=w759, index=w760) -> (element=w758:i32)
              n215 = case shown="28" w760 {
                tunnel: w759 -> [w764 w768 w773 w779 w783 w791 w795 w798 w803 w808 w816 w824 w831 w846 w860 w874 w888 w894]
                tunnel: [w764 w768 w773 w779 w783 w791 w795 w798 w803 w808 w816 w824 w831 w846 w860 w874 w888 w894] -> w763
                tunnel: [w765 w766 w771 w778 w784 w789 w794 w797 w802 w807 w815 w823 w829 w835 w849 w863 w877 w893] -> w762
                tunnel: w761 -> [w765 _ w771 w778 w784 w789 w794 w797 w802 w807 w815 w823 w829 w835 w849 w863 w877 w893]
                tunnel: w758 -> [_ w767 w770 w776 w782 w788 w793 w796 w800 w805 w813 w822 w828 w836 w850 w864 w878 w890]
                frame 0 {
                  # "SCHEDULE"
                }
                frame 1, Default {
                  n216 = call "Number-to-hex-2-digit.vi"("dec_num"=w767) -> ("hex_num"=w766:string)  [unwired: 10 in]
                }
                frame 2 {
                  # "HIGH1C"
                  n217 = call "Number-to-hex-2-digit.vi"("dec_num"=w770) -> ("hex_num"=w769:string)  [unwired: 10 in]
                  n218 = Concatenate Strings(w771, w769) -> (w774:string)
                  n219 = Hexadecimal String To Number(string=w774) -> (number=→"HI":u32)  [unwired: 2 in, 1 out]
                }
                frame 4 {
                  # "LOW1C"
                  n220 = call "Number-to-hex-2-digit.vi"("dec_num"=w776) -> ("hex_num"=w775:string)  [unwired: 10 in]
                  n221 = Concatenate Strings(w778, w775) -> (w780:string)
                  n222 = Hexadecimal String To Number(string=w780) -> (number=→"LO":u32)  [unwired: 2 in, 1 out]
                }
                frame 6 {
                  # "HIGH2C"
                  n223 = call "Number-to-hex-2-digit.vi"("dec_num"=w782) -> ("hex_num"=w781:string)  [unwired: 10 in]
                  n224 = Concatenate Strings(w784, w781) -> (w786:string)
                  n225 = Hexadecimal String To Number(string=w786) -> (number=→"High current #2 %":u32)  [unwired: 2 in, 1 out]
                }
                frame 8 {
                  # "LOW2C"
                  n226 = call "Number-to-hex-2-digit.vi"("dec_num"=w788) -> ("hex_num"=w787:string)  [unwired: 10 in]
                  n227 = Concatenate Strings(w789, w787) -> (w792:string)
                  n228 = Hexadecimal String To Number(string=w792) -> (number=→"Low current #2 %":u32)  [unwired: 2 in, 1 out]
                }
                frame 9 {
                  # "ANGLE LIMIT 1"
                  "HI" <- w793
                }
                frame 10 {
                  # "ANGLE LIMIT 2"
                  "Conduction limit #2" <- w796
                }
                frame 12 {
                  # "WELD COUNT LIMIT"
                  n229 = call "Number-to-hex-2-digit.vi"("dec_num"=w800) -> ("hex_num"=w799:string)  [unwired: 10 in]
                  n230 = Concatenate Strings(w802, w799) -> (w804:string)
                  n231 = Hexadecimal String To Number(string=w804) -> (number=→"Weld count limit":u32)  [unwired: 2 in, 1 out]
                }
                frame 13 {
                  # "START VALUE"
                  n232 = case shown="0, Default" w805 {
                    tunnel: ["MAINTAINED" "PULSED" "LATCHED" "SEAM"] -> w806
                    frame 0, Default {
                    }
                    frame 1 {
                    }
                    frame 2 {
                    }
                    frame 3 {
                    }
                  }
                  "Start value" <- w806
                  "Start value" <- w805
                }
                frame 14 {
                  # "WELD MODE"
                  n233 = case shown="1" w813 {
                    tunnel: ["SPOT" "REPEAT" "SUCCESSIVE" "CHANING"] -> w814
                    frame 0, Default {
                    }
                    frame 1 {
                    }
                    frame 2 {
                    }
                    frame 3 {
                    }
                  }
                  "Weld mode" <- w814
                  "Weld mode" <- w813
                }
                frame 16 {
                  # "LOP"
                  n234 = call "Number-to-hex-2-digit.vi"("dec_num"=w822) -> ("hex_num"=w821:string)  [unwired: 10 in]
                  n235 = Concatenate Strings(w823, w821) -> (w826:string)
                  n236 = Hexadecimal String To Number(string=w826) -> (number=→"LO":u32)  [unwired: 2 in, 1 out]
                }
                frame 18 {
                  # "HIP"
                  n237 = call "Number-to-hex-2-digit.vi"("dec_num"=w828) -> ("hex_num"=w827:string)  [unwired: 10 in]
                  n238 = Concatenate Strings(w829, w827) -> (w832:string)
                  n239 = Hexadecimal String To Number(string=w832) -> (number=→"HI":u32)  [unwired: 2 in, 1 out]
                }
                frame 20 {
                  # "VOLTHIW1"
                  n240 = call "Number-to-hex-2-digit.vi"("dec_num"=w836) -> ("hex_num"=w845:string)  [unwired: 10 in]
                  n241 = Concatenate Strings(w835, w845) -> (w837:string)
                  n242 = Hexadecimal String To Number(string=w837) -> (number=w838:u32)  [unwired: 2 in, 1 out]
                  n243 = Quotient & Remainder(x=w838, y=u32 100) -> (x-y*floor(x/y)=w840:u32, floor(x/y)=w841:u32)
                  n244 = Number To Decimal String(number=w841) -> (decimal integer string=w842:string)  [unwired: 1 in]
                  n245 = Number To Decimal String(number=w840) -> (decimal integer string=w844:string)  [unwired: 1 in]
                  n246 = Concatenate Strings(w842, "." ("string"), w844) -> (w834:string)
                  "HI" <- w834
                  n247 = Fract/Exp String To Number(string=w834) -> (number=→"VOLTHIW1":dbl)  [unwired: 3 in, 1 out]
                }
                frame 22 {
                  # "VOLTLOW1"
                  n248 = call "Number-to-hex-2-digit.vi"("dec_num"=w850) -> ("hex_num"=w859:string)  [unwired: 10 in]
                  n249 = Concatenate Strings(w849, w859) -> (w851:string)
                  n250 = Hexadecimal String To Number(string=w851) -> (number=w852:u32)  [unwired: 2 in, 1 out]
                  n251 = Quotient & Remainder(x=w852, y=u32 100) -> (x-y*floor(x/y)=w854:u32, floor(x/y)=w855:u32)
                  n252 = Number To Decimal String(number=w855) -> (decimal integer string=w856:string)  [unwired: 1 in]
                  n253 = Number To Decimal String(number=w854) -> (decimal integer string=w858:string)  [unwired: 1 in]
                  n254 = Concatenate Strings(w856, "." ("string"), w858) -> (w848:string)
                  "LO" <- w848
                  n255 = Fract/Exp String To Number(string=w848) -> (number=→"VOLTLOW1":dbl)  [unwired: 3 in, 1 out]
                }
                frame 24 {
                  # "VOLTHIW2"
                  n256 = call "Number-to-hex-2-digit.vi"("dec_num"=w864) -> ("hex_num"=w873:string)  [unwired: 10 in]
                  n257 = Concatenate Strings(w863, w873) -> (w865:string)
                  n258 = Hexadecimal String To Number(string=w865) -> (number=w866:u32)  [unwired: 2 in, 1 out]
                  n259 = Quotient & Remainder(x=w866, y=u32 100) -> (x-y*floor(x/y)=w868:u32, floor(x/y)=w869:u32)
                  n260 = Number To Decimal String(number=w869) -> (decimal integer string=w870:string)  [unwired: 1 in]
                  n261 = Number To Decimal String(number=w868) -> (decimal integer string=w872:string)  [unwired: 1 in]
                  n262 = Concatenate Strings(w870, "." ("string"), w872) -> (w862:string)
                  "VOLTHIW2" <- w862
                  n263 = Fract/Exp String To Number(string=w862) -> (number=→"VOLTHIW2":dbl)  [unwired: 3 in, 1 out]
                }
                frame 26 {
                  # "VOLTLOW2"
                  n264 = call "Number-to-hex-2-digit.vi"("dec_num"=w878) -> ("hex_num"=w887:string)  [unwired: 10 in]
                  n265 = Concatenate Strings(w877, w887) -> (w879:string)
                  n266 = Hexadecimal String To Number(string=w879) -> (number=w880:u32)  [unwired: 2 in, 1 out]
                  n267 = Quotient & Remainder(x=w880, y=u32 100) -> (x-y*floor(x/y)=w882:u32, floor(x/y)=w883:u32)
                  n268 = Number To Decimal String(number=w883) -> (decimal integer string=w884:string)  [unwired: 1 in]
                  n269 = Number To Decimal String(number=w882) -> (decimal integer string=w886:string)  [unwired: 1 in]
                  n270 = Concatenate Strings(w884, "." ("string"), w886) -> (w876:string)
                  "VOLTLOW2" <- w876
                  n271 = Fract/Exp String To Number(string=w876) -> (number=→"VOLTLOW2":dbl)  [unwired: 3 in, 1 out]
                }
                frame 28 {
                  # "FIRE"
                  n272 = call "Number-to-hex-2-digit.vi"("dec_num"=w890) -> ("hex_num"=w889:string)  [unwired: 10 in]
                  n273 = Concatenate Strings(w893, w889) -> (w892:string)
                  n274 = Hexadecimal String To Number(string=w892) -> (number=→"FIRE =":u32)  [unwired: 2 in, 1 out]
                }
              }
            }
          }
          frame "Load Read" {
            n275 = Index Array(array=w899, index=0) -> (element=→"Act. SCHE.":i32)
          }
          frame "Schedule Read" {
            n276 = for {
              N: 35 -> [_]
              shift-right: [w910] -> _
              shift-left: "" -> [w909]
              shift-right: [w908] -> _
              shift-left: w903 -> [w906]
              i -> [w907]
              n277 = Index Array(array=w906, index=w907) -> (element=w905:i32)
              n278 = case shown="34" w907 {
                tunnel: [w912 w913 w916 w922 w928 w937 w940 w946 w952 w962 w964 w970 w976 w982 w988 w1006 w1012 w1023 w1025 w1036] -> w910
                tunnel: w909 -> [w912 _ w916 w922 w928 w937 w940 w946 w952 w962 w964 w970 w976 w982 w988 w1006 w1012 w1023 w1025 w1036]
                tunnel: w906 -> [w911 w915 w921 w927 w933 w936 w945 w949 w956 w961 w969 w975 w981 w987 w993 w1007 w1021 w1024 w1030 w1037]
                tunnel: [w911 w915 w921 w927 w933 w936 w945 w949 w956 w961 w969 w975 w981 w987 w993 w1007 w1021 w1024 w1030 w1037] -> w908
                tunnel: w905 -> [_ w914 w918 w924 w930 w935 w942 w948 w954 w959 w966 w972 w978 w984 w990 w997 w1011 w1022 w1027 w1031]
                frame 0 {
                }
                frame 1, Default {
                  n279 = call "Number-to-hex-2-digit.vi"("dec_num"=w914) -> ("hex_num"=w913:string)  [unwired: 10 in]
                }
                frame 2 {
                  n280 = call "Number-to-hex-2-digit.vi"("dec_num"=w918) -> ("hex_num"=w917:string)  [unwired: 10 in]
                  n281 = Concatenate Strings(w916, w917) -> (w919:string)
                  n282 = Hexadecimal String To Number(string=w919) -> (number=→"SQD":u32)  [unwired: 2 in, 1 out]
                }
                frame 4 {
                  n283 = call "Number-to-hex-2-digit.vi"("dec_num"=w924) -> ("hex_num"=w923:string)  [unwired: 10 in]
                  n284 = Concatenate Strings(w922, w923) -> (w925:string)
                  n285 = Hexadecimal String To Number(string=w925) -> (number=→"SQZ":u32)  [unwired: 2 in, 1 out]
                }
                frame 6 {
                  n286 = call "Number-to-hex-2-digit.vi"("dec_num"=w930) -> ("hex_num"=w929:string)  [unwired: 10 in]
                  n287 = Concatenate Strings(w928, w929) -> (w932:string)
                  n288 = Hexadecimal String To Number(string=w932) -> (number=→"UP1":u32)  [unwired: 2 in, 1 out]
                }
                frame 8 {
                  n289 = call "Number-to-hex-2-digit.vi"("dec_num"=w935) -> ("hex_num"=w934:string)  [unwired: 10 in]
                  n290 = Concatenate Strings(w937, w934) -> (w939:string)
                  n291 = Hexadecimal String To Number(string=w939) -> (number=→"W1":u32)  [unwired: 2 in, 1 out]
                }
                frame 10 {
                  n292 = call "Number-to-hex-2-digit.vi"("dec_num"=w942) -> ("hex_num"=w941:string)  [unwired: 10 in]
                  n293 = Concatenate Strings(w940, w941) -> (w944:string)
                  n294 = Hexadecimal String To Number(string=w944) -> (number=→"DN1":u32)  [unwired: 2 in, 1 out]
                }
                frame 12 {
                  n295 = call "Number-to-hex-2-digit.vi"("dec_num"=w948) -> ("hex_num"=w947:string)  [unwired: 10 in]
                  n296 = Concatenate Strings(w946, w947) -> (w951:string)
                  n297 = Hexadecimal String To Number(string=w951) -> (number=→"CO":u32)  [unwired: 2 in, 1 out]
                }
                frame 14 {
                  n298 = call "Number-to-hex-2-digit.vi"("dec_num"=w954) -> ("hex_num"=w953:string)  [unwired: 10 in]
                  n299 = Concatenate Strings(w952, w953) -> (w955:string)
                  n300 = Hexadecimal String To Number(string=w955) -> (number=→"UP2":u32)  [unwired: 2 in, 1 out]
                }
                frame 16 {
                  n301 = call "Number-to-hex-2-digit.vi"("dec_num"=w959) -> ("hex_num"=w958:string)  [unwired: 10 in]
                  n302 = Concatenate Strings(w962, w958) -> (w963:string)
                  n303 = Hexadecimal String To Number(string=w963) -> (number=→"W2":u32)  [unwired: 2 in, 1 out]
                }
                frame 18 {
                  n304 = call "Number-to-hex-2-digit.vi"("dec_num"=w966) -> ("hex_num"=w965:string)  [unwired: 10 in]
                  n305 = Concatenate Strings(w964, w965) -> (w968:string)
                  n306 = Hexadecimal String To Number(string=w968) -> (number=→"DN2":u32)  [unwired: 2 in, 1 out]
                }
                frame 20 {
                  n307 = call "Number-to-hex-2-digit.vi"("dec_num"=w972) -> ("hex_num"=w971:string)  [unwired: 10 in]
                  n308 = Concatenate Strings(w970, w971) -> (w974:string)
                  n309 = Hexadecimal String To Number(string=w974) -> (number=→"HLD":u32)  [unwired: 2 in, 1 out]
                }
                frame 22 {
                  n310 = call "Number-to-hex-2-digit.vi"("dec_num"=w978) -> ("hex_num"=w977:string)  [unwired: 10 in]
                  n311 = Concatenate Strings(w976, w977) -> (w980:string)
                  n312 = Hexadecimal String To Number(string=w980) -> (number=→"OFF":u32)  [unwired: 2 in, 1 out]
                }
                frame 24 {
                  n313 = call "Number-to-hex-2-digit.vi"("dec_num"=w984) -> ("hex_num"=w983:string)  [unwired: 10 in]
                  n314 = Concatenate Strings(w982, w983) -> (w986:string)
                  n315 = Hexadecimal String To Number(string=w986) -> (number=→"%HEAT 1":u32)  [unwired: 2 in, 1 out]
                }
                frame 26 {
                  n316 = call "Number-to-hex-2-digit.vi"("dec_num"=w990) -> ("hex_num"=w989:string)  [unwired: 10 in]
                  n317 = Concatenate Strings(w988, w989) -> (w992:string)
                  n318 = Hexadecimal String To Number(string=w992) -> (number=→"%HEAT 2":u32)  [unwired: 2 in, 1 out]
                }
                frame 28 {
                  n319 = call "Number-to-hex-2-digit.vi"("dec_num"=w997) -> ("hex_num"=w996:string)  [unwired: 10 in]
                  n320 = Concatenate Strings(w1006, w996) -> (w1005:string)
                  n321 = Hexadecimal String To Number(string=w1005) -> (number=w1004:u32)  [unwired: 2 in, 1 out]
                  n322 = Quotient & Remainder(x=w1004, y=u32 100) -> (x-y*floor(x/y)=w1002:u32, floor(x/y)=w1001:u32)
                  n323 = Number To Decimal String(number=w1001) -> (decimal integer string=w1000:string)  [unwired: 1 in]
                  n324 = Number To Decimal String(number=w1002) -> (decimal integer string=w998:string)  [unwired: 1 in]
                  n325 = Concatenate Strings(w1000, "." ("string"), w998) -> (w995:string)
                  "CURRENT #1" <- w995
                  n326 = Fract/Exp String To Number(string=w995) -> (number=→"CURRENT #1":dbl)  [unwired: 3 in, 1 out]
                }
                frame 30 {
                  n327 = call "Number-to-hex-2-digit.vi"("dec_num"=w1011) -> ("hex_num"=w1010:string)  [unwired: 10 in]
                  n328 = Concatenate Strings(w1012, w1010) -> (w1020:string)
                  n329 = Hexadecimal String To Number(string=w1020) -> (number=w1019:u32)  [unwired: 2 in, 1 out]
                  n330 = Quotient & Remainder(x=w1019, y=u32 100) -> (x-y*floor(x/y)=w1017:u32, floor(x/y)=w1016:u32)
                  n331 = Number To Decimal String(number=w1016) -> (decimal integer string=w1015:string)  [unwired: 1 in]
                  n332 = Number To Decimal String(number=w1017) -> (decimal integer string=w1013:string)  [unwired: 1 in]
                  n333 = Concatenate Strings(w1015, "." ("string"), w1013) -> (w1009:string)
                  "CURRENT #2" <- w1009
                  n334 = Fract/Exp String To Number(string=w1009) -> (number=→"CURRENT #2":dbl)  [unwired: 3 in, 1 out]
                }
                frame 31 {
                  "IMPULSE" <- w1022
                }
                frame 33 {
                  n335 = call "Number-to-hex-2-digit.vi"("dec_num"=w1027) -> ("hex_num"=w1026:string)  [unwired: 10 in]
                  n336 = Concatenate Strings(w1025, w1026) -> (w1028:string)
                  n337 = Hexadecimal String To Number(string=w1028) -> (number=→"FORCE":u32)  [unwired: 2 in, 1 out]
                }
                frame 34 {
                  n338 = Get Date/Time String() -> (date string=w1035:string, time string=w1032:string)  [unwired: 3 in]
                  n339 = Concatenate Strings(w1035, " a la(s)" ("string"), w1032) -> (→"Última vez actualizado":string)
                  "FORCE CHANNEL" <- w1031
                }
              }
            }
          }
          frame "Status Read" {
            n340 = for {
              N: 9 -> [_]
              shift-right: [w1060] -> _
              shift-left: w1047 -> [w1056]
              shift-right: [w1059] -> _
              shift-left: "" -> [w1061]
              shift-right: [w1049] -> _
              shift-left: FALSE -> [w1058]
              shift-right: [w1053] -> _
              shift-left: u32 6618880 ("STATUS") -> [w1054]
              shift-right: [w1052] -> w1042
              shift-left: 0 -> [w1051]
              i -> [w1057]
              n341 = Index Array(array=w1056, index=w1057) -> (element=w1055:i32)
              n342 = case shown="3" w1057 {
                tunnel: w1056 -> [w1065 w1077 w1094 w1103 w1107 w1110 w1115 w1190]
                tunnel: w1061 -> [_ w1076 w1093 w1102 w1106 w1109 w1114 w1191]
                tunnel: [w1065 w1077 w1094 w1103 w1107 w1110 w1115 w1190] -> w1060
                tunnel: [w1064 w1076 w1093 w1102 w1106 w1109 w1114 w1191] -> w1059
                tunnel: [_ w1069 w1086 _ _ _ _ _] -> w1049
                tunnel: w1058 -> [_ _ _ _ _ _ _ _]
                tunnel: w1055 -> [w1063 w1071 w1088 w1100 w1105 w1108 w1113 w1189]
                tunnel: w1054 -> [w1062 w1068 w1085 _ _ _ _ _]
                tunnel: [w1062 w1067 w1083 _ _ _ _ _] -> w1053
                frame 0, Default {
                  n343 = call "Number-to-hex-2-digit.vi"("dec_num"=w1063) -> ("hex_num"=w1064:string)  [unwired: 10 in]
                }
                frame 1 {
                  # "Major Error Bit Pattern, son 12 bits con un error identificador cada uno"
                  # "Identifica que soldadora fue"
                  # "Identifica el error"
                  n344 = call "Number-to-hex-2-digit.vi"("dec_num"=w1071) -> ("hex_num"=w1070:string)  [unwired: 10 in]
                  n345 = Concatenate Strings(w1076, w1070) -> (w1078:string)
                  n346 = Hexadecimal String To Number(string=w1078) -> (number=w1075:u32)  [unwired: 2 in, 1 out]
                  n347 = And(x=w1075, y=u32 4095) -> (x .and. y?=w1073:u32)
                  n348 = case shown="16" w1073 {
                    frame 0 {
                    }
                    frame 1 {
                      n349 = call "Display Message to User11"() -> ()  [unwired: 10 in, 2 out]
                    }
                    frame 2 {
                      n350 = call "Display Message to User12"() -> ()  [unwired: 10 in, 2 out]
                    }
                    frame 4 {
                      n351 = call "Display Message to User13"() -> ()  [unwired: 10 in, 2 out]
                    }
                    frame 8 {
                      n352 = call "Display Message to User14"() -> ()  [unwired: 10 in, 2 out]
                    }
                    frame 16 {
                    }
                    frame 32 {
                      n353 = call "Display Message to User15"() -> ()  [unwired: 10 in, 2 out]
                    }
                    frame 64 {
                      n354 = call "Display Message to User16"() -> ()  [unwired: 10 in, 2 out]
                    }
                    frame 128 {
                      n355 = call "Display Message to User17"() -> ()  [unwired: 10 in, 2 out]
                    }
                    frame 256 {
                      n356 = call "Display Message to User18"() -> ()  [unwired: 10 in, 2 out]
                    }
                    frame 512 {
                      n357 = call "Display Message to User19"() -> ()  [unwired: 10 in, 2 out]
                    }
                    frame 1024 {
                    }
                    frame 2048 {
                      n358 = call "Display Message to User20"() -> ()  [unwired: 10 in, 2 out]
                    }
                    frame 9999, Default {
                    }
                  }
                  n359 = Not Equal?(x=w1073, y=u32 0) -> (x != y?=w1066:bool)
                  "sold1_error_fromLV" <- w1066
                  n360 = case shown="False" w1066 {
                    selector: w1066 -> [w1080 w1082]
                    tunnel: [w1080 w1082] -> w1069
                    tunnel: w1068 -> [w1079 _]
                    tunnel: [w1079 u32 16711680 ("STATUS")] -> w1067
                    frame False {
                    }
                    frame True {
                    }
                  }
                }
                frame 3 {
                  # "Minor Error Bit Pattern, son 13 bits con un error identificador cada uno"
                  n361 = call "Number-to-hex-2-digit.vi"("dec_num"=w1088) -> ("hex_num"=w1087:string)  [unwired: 10 in]
                  n362 = Concatenate Strings(w1093, w1087) -> (w1095:string)
                  n363 = Hexadecimal String To Number(string=w1095) -> (number=w1092:u32)  [unwired: 2 in, 1 out]
                  n364 = And(x=w1092, y=u32 8191) -> (x .and. y?=w1090:u32)
                  n365 = case shown="8" w1090 {
                    frame 0 {
                    }
                    frame 1 {
                    }
                    frame 2 {
                    }
                    frame 4 {
                      n366 = call "Display Message to User21"() -> ()  [unwired: 10 in, 2 out]
                    }
                    frame 8 {
                      n367 = call "Display Message to User22"() -> ()  [unwired: 10 in, 2 out]
                    }
                    frame 16 {
                    }
                    frame 32 {
                    }
                    frame 64 {
                    }
                    frame 128 {
                      n368 = call "Display Message to User23"() -> ()  [unwired: 10 in, 2 out]
                    }
                    frame 256 {
                      n369 = call "Display Message to User24"() -> ()  [unwired: 10 in, 2 out]
                    }
                    frame 512 {
                    }
                    frame 1024 {
                      n370 = call "Display Message to User25"() -> ()  [unwired: 10 in, 2 out]
                    }
                    frame 2048 {
                    }
                    frame 4096 {
                    }
                    frame 5555, Default {
                    }
                  }
                  n371 = Not Equal?(x=w1090, y=u32 0) -> (x != y?=w1084:bool)
                  "sold1_warning_fromLV" <- w1084
                  n372 = case shown="False" w1084 {
                    selector: w1084 -> [w1097 w1098]
                    tunnel: [w1097 w1098] -> w1086
                    tunnel: [w1096 u32 16772882 ("STATUS")] -> w1083
                    tunnel: w1085 -> [w1096 _]
                    frame False {
                    }
                    frame True {
                    }
                  }
                  "STATUS" <- w1083
                }
                frame 4 {
                  n373 = call "Number-to-hex-2-digit.vi"("dec_num"=w1100) -> ("hex_num"=w1101:string)  [unwired: 10 in]
                  n374 = Hexadecimal String To Number(string=w1101) -> ()  [unwired: 2 in, 2 out]
                }
                frame 5 {
                  n375 = call "Number-to-hex-2-digit.vi"("dec_num"=w1105) -> ("hex_num"=w1104:string)  [unwired: 10 in]
                  n376 = Hexadecimal String To Number(string=w1104) -> ()  [unwired: 2 in, 2 out]
                }
                frame 6 {
                  n377 = case shown="0, Default" w1108 {
                    tunnel: ["No change" "Change"] -> _
                    frame 0, Default {
                    }
                    frame 1 {
                    }
                  }
                }
                frame 7 {
                  n378 = case shown="21" w1113 {
                    tunnel: ["UNKNOWN" "1. Run screen" "2. Stepper screen" "3. Weld mode screen" "4. % heat monitor screen" "5. Valve screen for 12 valves" "6. Not used" "7. Program screen for constant current modes" "8. System values screen" "9. Linked schedules screen" "10. Not used" "11. Not used" "12. Duplicate starting schedules in link lists screen." "13. Scchedule programming screen" "14. Not used" "15. Hidden screen" "16. Copy schedule screen" "17. System valve screen - 4 valve option" "18. System valve screen - 12 valve option" "19. Full current error screen" "20. Weld 1 current greater than full current error screen" "21. Weld 2 current greater than full current error screen" "22. Weld 1 current less than 20% of full current error screen" "23. Weld 2 current less than 20% of full current error screen" "24. Weld monitor screen - constant current modes" "25. Valve screen - 4 valves" "26. Weld monitor programming screen" "27. Weld 1 current plus stepper value exceeds full current screen." "28. Weld 2 current plus stepper value exceeds full current screen." "29. Emergency stop screen" "30. Thermostat over temperature screen" "31. No current error screen" "32. Full wave conduction angles reached error screen" "33. Mode change error screen" "34. Weld 1 current too high" "35. Weld 2 current too high" "Weld 1 current too low" "Weld 2 current too low" "38. Weld 1 conduction angle too high" "39. Weld 2 conduction angle too high" "40. Step count too high error screen" "41. Modified schedule not saved error screen" "42. Duplicate SCR number assigned error screen" "43. Weld count reached limit error screen" "44. Stepper end reached error screen." "45. Not used" "46. Simplified schedule screen" "47. Simple %heat screen" "48. Not used" "49. Seam weld in primary current control screen" "50. Seam weld in %heat mode screen." "51. Seam weld simplified screen - constant current modes" "52. Seam weld simplified screen - %heat modes" "53. SCR shorted screen." "54. List of boards installed screen." "55. Low line voltage screen." "56. High line voltage screen" "57. Current scaling error" "58. Not used" "59. Continuous seam weld enabled mode screen." "60. Roll spot weld enabled mode screen" "61. Schedule number error screen" "62. System values continuation screen" "63. Schedule W1 and W2 times set to 0 error screen" "Pixel test info screen" "65. Not used" "66. Not used" "67. Second hidden screen" "68. Incorrect SCR number detected screen" "69. Pressure switch error" "70. Force calibration screen" "71. System boot-up screen"] -> _
                    frame 0, Default {
                    }
                    frame 1 {
                    }
                    frame 2 {
                    }
                    frame 3 {
                    }
                    frame 4 {
                    }
                    frame 5 {
                    }
                    frame 6 {
                    }
                    frame 7 {
                    }
                    frame 8 {
                    }
                    frame 9 {
                    }
                    frame 10 {
                    }
                    frame 11 {
                    }
                    frame 12 {
                    }
                    frame 13 {
                    }
                    frame 14 {
                    }
                    frame 15 {
                    }
                    frame 16 {
                    }
                    frame 17 {
                    }
                    frame 18 {
                    }
                    frame 19 {
                    }
                    frame 20 {
                    }
                    frame 21 {
                    }
                    frame 22 {
                    }
                    frame 23 {
                    }
                    frame 24 {
                    }
                    frame 25 {
                    }
                    frame 26 {
                    }
                    frame 27 {
                    }
                    frame 28 {
                    }
                    frame 29 {
                    }
                    frame 30 {
                    }
                    frame 31 {
                    }
                    frame 32 {
                    }
                    frame 33 {
                    }
                    frame 34 {
                    }
                    frame 35 {
                    }
                    frame 36 {
                    }
                    frame 37 {
                    }
                    frame 38 {
                    }
                    frame 39 {
                    }
                    frame 40 {
                    }
                    frame 41 {
                    }
                    frame 42 {
                    }
                    frame 43 {
                    }
                    frame 44 {
                    }
                    frame 45 {
                    }
                    frame 46 {
                    }
                    frame 47 {
                    }
                    frame 48 {
                    }
                    frame 49 {
                    }
                    frame 50 {
                    }
                    frame 51 {
                    }
                    frame 52 {
                    }
                    frame 53 {
                    }
                    frame 54 {
                    }
                    frame 55 {
                    }
                    frame 56 {
                    }
                    frame 57 {
                    }
                    frame 58 {
                    }
                    frame 59 {
                    }
                    frame 60 {
                    }
                    frame 61 {
                    }
                    frame 62 {
                    }
                    frame 63 {
                    }
                    frame 64 {
                    }
                    frame 65 {
                    }
                    frame 66 {
                    }
                    frame 67 {
                    }
                    frame 68 {
                    }
                    frame 69 {
                    }
                    frame 70 {
                    }
                    frame 71 {
                    }
                  }
                }
                frame 8 {
                  n379 = call "Number-to-hex-2-digit.vi"("dec_num"=w1189) -> ("hex_num"=w1188:string)  [unwired: 10 in]
                  n380 = Hexadecimal String To Number(string=w1188) -> ()  [unwired: 2 in, 2 out]
                }
              }
              n381 = Boolean To (0,1)(Boolean=w1049) -> (0, 1=w1050:i16)
              n382 = Add(x=w1050, y=w1051) -> (x+y=w1052:i32)
            }
            n383 = Equal?(x=w1042, y=0) -> (x = y?=w1040:bool)
            n384 = Get Date/Time In Seconds() -> (seconds since 1Jan1904=→"current time":timestamp)
          }
          frame "System Read" {
            n385 = for {
              N: 25 -> [_]
              shift-right: [w1238] -> _
              shift-left: w1233 -> [w1236]
              i -> [w1237]
              n386 = Index Array(array=w1236, index=w1237) -> (element=w1235:i32)
              n387 = case shown="15" w1237 {
                tunnel: [w1239 w1240 w1241 w1243 w1247 w1251 w1255 w1259 w1263 w1266 w1268 w1275 w1279 w1286 w1294 w1300 w1308 w1312 w1316 w1320 w1325 w1329 w1332 w1334 w1342] -> w1238
                tunnel: w1236 -> [w1239 w1240 w1241 w1243 w1247 w1251 w1255 w1259 w1263 w1266 w1268 w1275 w1279 w1286 w1294 w1300 w1308 w1312 w1316 w1320 w1325 w1329 w1332 w1334 w1342]
                tunnel: w1235 -> [_ _ _ w1242 w1246 w1250 w1254 w1258 w1262 _ w1267 w1274 w1278 w1285 w1293 w1299 w1307 w1311 w1315 w1319 w1324 w1328 _ w1333 w1338]
                frame 0, Default {
                }
                frame 1 {
                }
                frame 2 {
                }
                frame 3 {
                  n388 = case shown="0, Default" w1242 {
                    tunnel: ["OFF" "ON"] -> _
                    frame 0, Default {
                    }
                    frame 1 {
                    }
                  }
                }
                frame 4 {
                  n389 = case shown="0, Default" w1246 {
                    tunnel: ["OFF" "ON"] -> _
                    frame 0, Default {
                    }
                    frame 1 {
                    }
                  }
                }
                frame 5 {
                  n390 = case shown="1" w1250 {
                    tunnel: ["OFF" "ON"] -> _
                    frame 0, Default {
                    }
                    frame 1 {
                    }
                  }
                }
                frame 6 {
                  n391 = case shown="0, Default" w1254 {
                    tunnel: ["OFF" "ON"] -> _
                    frame 0, Default {
                    }
                    frame 1 {
                    }
                  }
                }
                frame 7 {
                  n392 = case shown="1" w1258 {
                    tunnel: ["OFF" "ON"] -> _
                    frame 0, Default {
                    }
                    frame 1 {
                    }
                  }
                }
                frame 8 {
                  n393 = case shown="0, Default" w1262 {
                    tunnel: ["OFF" "ON"] -> _
                    frame 0, Default {
                    }
                    frame 1 {
                    }
                  }
                }
                frame 9 {
                }
                frame 10 {
                  n394 = case shown="2" w1267 {
                    tunnel: ["Primary c. current" "% Heat primary" "Secondary c. current" "%Heat secondary" "% Heat"] -> _
                    frame 0, Default {
                    }
                    frame 1 {
                    }
                    frame 2 {
                    }
                    frame 3 {
                    }
                    frame 4 {
                    }
                  }
                }
                frame 11 {
                  n395 = case shown="1" w1274 {
                    tunnel: ["Two Stage" "One Stage"] -> _
                    frame 0, Default {
                    }
                    frame 1 {
                    }
                  }
                }
                frame 12 {
                  n396 = case shown="1" w1278 {
                    tunnel: ["Spot" "Continuous seam" "Roll spot"] -> _
                    frame 0, Default {
                    }
                    frame 1 {
                    }
                    frame 2 {
                    }
                  }
                }
                frame 13 {
                  n397 = case shown="1" w1285 {
                    tunnel: ["Local" "Remote"] -> _
                    tunnel: [TRUE FALSE] -> w1284
                    tunnel: [FALSE TRUE] -> w1283
                    frame 0, Default {
                    }
                    frame 1 {
                    }
                  }
                  "Local" <- w1284
                  "Remote" <- w1283
                }
                frame 14 {
                  n398 = case shown="1" w1293 {
                    tunnel: ["OFF" "ON"] -> _
                    frame 0, Default {
                    }
                    frame 1 {
                    }
                  }
                }
                frame 15 {
                  n399 = case shown="0, Default" w1299 {
                    tunnel: ["Local" "Host"] -> _
                    tunnel: [TRUE FALSE] -> w1298
                    tunnel: [FALSE TRUE] -> w1297
                    frame 0, Default {
                    }
                    frame 1 {
                    }
                  }
                  "Panel (Local)" <- w1298
                  "PC (Remote)" <- w1297
                }
                frame 16 {
                  n400 = case shown="0, Default" w1307 {
                    tunnel: ["Maintained" "Pulsed"] -> _
                    frame 0, Default {
                    }
                    frame 1 {
                    }
                  }
                }
                frame 17 {
                  n401 = case shown="0, Default" w1311 {
                    tunnel: ["OFF" "ON"] -> _
                    frame 0, Default {
                    }
                    frame 1 {
                    }
                  }
                }
                frame 18 {
                  n402 = case shown="0, Default" w1315 {
                    tunnel: ["OFF" "ON"] -> _
                    frame 0, Default {
                    }
                    frame 1 {
                    }
                  }
                }
                frame 19 {
                  n403 = case shown="2" w1319 {
                    tunnel: ["OFF" "F1" "F1 - F8"] -> _
                    frame 0, Default {
                    }
                    frame 1 {
                    }
                    frame 2 {
                    }
                  }
                }
                frame 20 {
                  n404 = case shown="1" w1324 {
                    tunnel: ["PEAK" "RMS"] -> _
                    frame 0, Default {
                    }
                    frame 1 {
                    }
                  }
                }
                frame 21 {
                  n405 = case shown="1" w1328 {
                    tunnel: ["W1/W2" "Last cycle"] -> _
                    frame 0, Default {
                    }
                    frame 1 {
                    }
                  }
                }
                frame 22 {
                }
                frame 23 {
                  n406 = case shown="0, Default" w1333 {
                    tunnel: ["NONE" "PRI" "SEC"] -> _
                    frame 0, Default {
                    }
                    frame 1 {
                    }
                    frame 2 {
                    }
                  }
                }
                frame 24 {
                  n407 = Get Date/Time String() -> (date string=w1341:string, time string=w1339:string)  [unwired: 3 in]
                  n408 = case shown="1" w1338 {
                    tunnel: ["60" "50"] -> _
                    frame 0, Default {
                    }
                    frame 1 {
                    }
                  }
                  n409 = Concatenate Strings(w1341, " a la(s)" ("string"), w1339) -> ()  [unwired: 1 out]
                }
              }
            }
            n410 = local read "SCHEDULE"() -> (w1212:i32)
            n411 = local write "SCHEDULE"(w1212) -> ()
            n412 = local read "Conduction limit #2"() -> (w1227:dbl)
            n413 = local read "High current #2 %"() -> (w1229:dbl)
            n414 = local read "Low current #2 %"() -> (w1219:dbl)
            n415 = local read "Weld count limit"() -> (w1226:dbl)
            n416 = local read "VOLTLOW1"() -> (w1218:dbl)
            n417 = local read "VOLTLOW2"() -> (w1216:dbl)
            n418 = local read "Weld mode"() -> (w1224:i32)
            n419 = local read "VOLTHIW1"() -> (w1221:dbl)
            n420 = local read "VOLTHIW2"() -> (w1217:dbl)
            n421 = local read "Start value"() -> (w1225:i32)
            n422 = local read "FIRE ="() -> (w1215:u32)
            n423 = local read "LO"() -> (w1223:dbl)
            n424 = local read "LO"() -> (w1220:dbl)
            n425 = local read "HI"() -> (w1222:dbl)
            n426 = local read "HI"() -> (w1230:dbl)
            n427 = local read "HI"() -> (w1228:dbl)
            n428 = local read "MONITOR SET"() -> (w1232:T9)
            n429 = Bundle(cluster=w1232, "HIGH1C"=w1230, "W1"=w1220, "HIGH2C"=w1229, "W2"=w1219, "ANGLE 1"=w1228, "ANGLE 2"=w1227, "Weld count limit"=w1226, "Start value"=w1225, "Weld mode"=w1224, "LOP"=w1223, "HIP"=w1222, "VOLTHIW1"=w1221, "VOLTLOW1"=w1218, "VOLTHIW2"=w1217, "VOLTLOW2"=w1216, "FIRE ="=w1215) -> (w1231:T9)
            n430 = local write "MONITOR SET"(w1231) -> ()
            n431 = local read "FORCE CHANNEL"() -> (w1194:dbl)
            n432 = local read "CURRENT #1"() -> (w1198:dbl)
            n433 = local read "CURRENT #2"() -> (w1197:dbl)
            n434 = local read "%HEAT 1"() -> (w1200:u32)
            n435 = local read "%HEAT 2"() -> (w1199:u32)
            n436 = local read "IMPULSE"() -> (w1196:dbl)
            n437 = local read "FORCE"() -> (w1195:dbl)
            n438 = local read "SQD"() -> (w1211:dbl)
            n439 = local read "DN1"() -> (w1207:dbl)
            n440 = local read "DN2"() -> (w1203:dbl)
            n441 = local read "HLD"() -> (w1202:dbl)
            n442 = local read "SQZ"() -> (w1210:dbl)
            n443 = local read "UP1"() -> (w1209:dbl)
            n444 = local read "UP2"() -> (w1205:dbl)
            n445 = local read "OFF"() -> (w1201:dbl)
            n446 = local read "W1"() -> (w1208:dbl)
            n447 = local read "CO"() -> (w1206:dbl)
            n448 = local read "W2"() -> (w1204:dbl)
            n449 = local read "SCHEDULE SET"() -> (w1214:T8)
            n450 = Bundle(cluster=w1214, "SQD"=w1211, "SQZ"=w1210, "UP1"=w1209, "W1"=w1208, "DN1"=w1207, "CO"=w1206, "UP2"=w1205, "W2"=w1204, "DN2"=w1203, "HLD"=w1202, "OFF"=w1201, "%HEAT 1"=w1200, "%HEAT 2"=w1199, "CURRENT #1"=w1198, "CURRENT #2"=w1197, "IMPULSE"=w1196, "FORCE"=w1195, "FORCE CHANNEL"=w1194) -> (w1213:T8)
            n451 = local write "SCHEDULE SET"(w1213) -> ()
          }
          frame "Report Read" {
            n452 = for {
              N: 30 -> [_]
              shift-right: [w1353] -> _
              shift-left: w1348 -> [w1354]
              shift-right: [w1350] -> _
              shift-left: "" -> [w1351]
              i -> [w1355]
              n453 = case shown="20" w1355 {
                selector: w1355 -> [w1358 w1365 w1375 w1387 w1400 w1412 w1424 w1436 w1448 w1460 w1472 w1484 w1496 w1508 w1520 w1532 w1544 w1556 w1568 w1580 w1593 w1604 w1615 w1627 w1640 w1653 w1665 w1677 w1690 w1706]
                tunnel: w1354 -> [w1357 w1359 w1374 w1384 w1398 w1410 w1422 w1434 w1445 w1458 w1471 w1481 w1494 w1507 w1518 w1531 w1542 w1555 w1567 w1578 w1592 w1603 w1613 w1626 w1639 w1650 w1664 w1676 w1686 w1705]
                tunnel: [w1357 w1359 w1374 w1384 w1398 w1410 w1422 w1434 w1445 w1458 w1471 w1481 w1494 w1507 w1518 w1531 w1542 w1555 w1567 w1578 w1592 w1603 w1613 w1626 w1639 w1650 w1664 w1676 w1686 w1705] -> w1353
                tunnel: 15 ("y") -> [_ w1363 w1370 w1383 w1396 w1411 w1421 w1433 w1447 w1459 w1468 w1483 w1495 w1505 w1519 w1530 w1543 w1554 w1566 w1579 w1591 w1602 w1614 w1625 w1638 w1651 w1663 w1673 w1689 w1702]
                tunnel: [w1356 w1360 w1371 w1386 w1397 w1409 w1420 w1435 w1444 w1457 w1469 w1482 w1492 w1506 w1516 w1529 w1540 w1553 w1564 w1577 w1589 w1601 w1612 w1623 w1637 w1649 w1662 w1674 w1687 w1703] -> w1350
                tunnel: w1351 -> [w1356 _ w1372 w1385 w1399 _ w1423 _ w1446 _ w1470 _ w1493 _ w1517 _ w1541 _ w1565 _ w1589 _ _ w1623 w1636 w1652 _ w1675 w1688 w1704]
                frame 0, Default {
                  n454 = Index Array(array=w1357, index=w1358) -> ()  [unwired: 1 out]
                }
                frame 1 {
                  n455 = Index Array(array=w1359, index=w1365) -> (element=w1362:i32)
                  n456 = Number To Hexadecimal String(2:w1362) -> (0:w1364:string)  [unwired: 1 in]
                  n457 = Less Or Equal?(x=w1362, y=w1363) -> (x <= y?=w1361:bool)
                  n458 = case shown="True" w1361 {
                    tunnel: [w1366 w1369] -> w1360
                    tunnel: w1364 -> [w1366 w1367]
                    frame False {
                    }
                    frame True {
                      n459 = Concatenate Strings("0" ("string"), w1367) -> (w1369:string)
                    }
                  }
                }
                frame 2 {
                  n460 = Index Array(array=w1374, index=w1375) -> (element=w1377:i32)
                  n461 = Number To Hexadecimal String(2:w1377) -> (0:w1378:string)  [unwired: 1 in]
                  n462 = Less Or Equal?(x=w1377, y=w1370) -> (x <= y?=w1376:bool)
                  n463 = case shown="True" w1376 {
                    tunnel: [w1379 w1382] -> w1373
                    tunnel: w1378 -> [w1379 w1380]
                    frame False {
                    }
                    frame True {
                      n464 = Concatenate Strings("0" ("string"), w1380) -> (w1382:string)
                    }
                  }
                  n465 = Concatenate Strings(w1372, w1373) -> (w1371:string)
                }
                frame 3 {
                  n466 = Index Array(array=w1384, index=w1387) -> (element=w1390:i32)
                  n467 = Number To Hexadecimal String(2:w1390) -> (0:w1391:string)  [unwired: 1 in]
                  n468 = Less Or Equal?(x=w1390, y=w1383) -> (x <= y?=w1389:bool)
                  n469 = case shown="True" w1389 {
                    tunnel: [w1392 w1395] -> w1388
                    tunnel: w1391 -> [w1392 w1393]
                    frame False {
                    }
                    frame True {
                      n470 = Concatenate Strings("0" ("string"), w1393) -> (w1395:string)
                    }
                  }
                  n471 = Concatenate Strings(w1385, w1388) -> (w1386:string)
                }
                frame 4 {
                  n472 = Index Array(array=w1398, index=w1400) -> (element=w1403:i32)
                  n473 = Number To Hexadecimal String(2:w1403) -> (0:w1404:string)  [unwired: 1 in]
                  n474 = Less Or Equal?(x=w1403, y=w1396) -> (x <= y?=w1402:bool)
                  n475 = case shown="True" w1402 {
                    tunnel: [w1405 w1408] -> w1401
                    tunnel: w1404 -> [w1405 w1406]
                    frame False {
                    }
                    frame True {
                      n476 = Concatenate Strings("0" ("string"), w1406) -> (w1408:string)
                    }
                  }
                  n477 = Concatenate Strings(w1399, w1401) -> (w1397:string)
                  n478 = Hexadecimal String To Number(string=w1397) -> ()  [unwired: 2 in, 2 out]
                }
                frame 5 {
                  n479 = Index Array(array=w1410, index=w1412) -> (element=w1414:i32)
                  n480 = Number To Hexadecimal String(2:w1414) -> (0:w1415:string)  [unwired: 1 in]
                  n481 = Less Or Equal?(x=w1414, y=w1411) -> (x <= y?=w1413:bool)
                  n482 = case shown="True" w1413 {
                    tunnel: [w1416 w1419] -> w1409
                    tunnel: w1415 -> [w1416 w1417]
                    frame False {
                    }
                    frame True {
                      n483 = Concatenate Strings("0" ("string"), w1417) -> (w1419:string)
                    }
                  }
                }
                frame 6 {
                  n484 = Index Array(array=w1422, index=w1424) -> (element=w1427:i32)
                  n485 = Number To Hexadecimal String(2:w1427) -> (0:w1428:string)  [unwired: 1 in]
                  n486 = Less Or Equal?(x=w1427, y=w1421) -> (x <= y?=w1426:bool)
                  n487 = case shown="True" w1426 {
                    tunnel: [w1429 w1432] -> w1425
                    tunnel: w1428 -> [w1429 w1430]
                    frame False {
                    }
                    frame True {
                      n488 = Concatenate Strings("0" ("string"), w1430) -> (w1432:string)
                    }
                  }
                  n489 = Concatenate Strings(w1423, w1425) -> (w1420:string)
                  n490 = Hexadecimal String To Number(string=w1420) -> ()  [unwired: 2 in, 2 out]
                }
                frame 7 {
                  n491 = Index Array(array=w1434, index=w1436) -> (element=w1438:i32)
                  n492 = Number To Hexadecimal String(2:w1438) -> (0:w1439:string)  [unwired: 1 in]
                  n493 = Less Or Equal?(x=w1438, y=w1433) -> (x <= y?=w1437:bool)
                  n494 = case shown="True" w1437 {
                    tunnel: [w1440 w1443] -> w1435
                    tunnel: w1439 -> [w1440 w1441]
                    frame False {
                    }
                    frame True {
                      n495 = Concatenate Strings("0" ("string"), w1441) -> (w1443:string)
                    }
                  }
                }
                frame 8 {
                  n496 = Index Array(array=w1445, index=w1448) -> (element=w1451:i32)
                  n497 = Number To Hexadecimal String(2:w1451) -> (0:w1452:string)  [unwired: 1 in]
                  n498 = Less Or Equal?(x=w1451, y=w1447) -> (x <= y?=w1450:bool)
                  n499 = case shown="True" w1450 {
                    tunnel: [w1453 w1456] -> w1449
                    tunnel: w1452 -> [w1453 w1454]
                    frame False {
                    }
                    frame True {
                      n500 = Concatenate Strings("0" ("string"), w1454) -> (w1456:string)
                    }
                  }
                  n501 = Concatenate Strings(w1446, w1449) -> (w1444:string)
                  n502 = Hexadecimal String To Number(string=w1444) -> ()  [unwired: 2 in, 2 out]
                }
                frame 9 {
                  n503 = Index Array(array=w1458, index=w1460) -> (element=w1462:i32)
                  n504 = Number To Hexadecimal String(2:w1462) -> (0:w1463:string)  [unwired: 1 in]
                  n505 = Less Or Equal?(x=w1462, y=w1459) -> (x <= y?=w1461:bool)
                  n506 = case shown="True" w1461 {
                    tunnel: [w1464 w1467] -> w1457
                    tunnel: w1463 -> [w1464 w1465]
                    frame False {
                    }
                    frame True {
                      n507 = Concatenate Strings("0" ("string"), w1465) -> (w1467:string)
                    }
                  }
                }
                frame 10 {
                  n508 = Index Array(array=w1471, index=w1472) -> (element=w1475:i32)
                  n509 = Number To Hexadecimal String(2:w1475) -> (0:w1476:string)  [unwired: 1 in]
                  n510 = Less Or Equal?(x=w1475, y=w1468) -> (x <= y?=w1474:bool)
                  n511 = case shown="True" w1474 {
                    tunnel: [w1477 w1480] -> w1473
                    tunnel: w1476 -> [w1477 w1478]
                    frame False {
                    }
                    frame True {
                      n512 = Concatenate Strings("0" ("string"), w1478) -> (w1480:string)
                    }
                  }
                  n513 = Concatenate Strings(w1470, w1473) -> (w1469:string)
                  n514 = Hexadecimal String To Number(string=w1469) -> ()  [unwired: 2 in, 2 out]
                }
                frame 11 {
                  n515 = Index Array(array=w1481, index=w1484) -> (element=w1486:i32)
                  n516 = Number To Hexadecimal String(2:w1486) -> (0:w1487:string)  [unwired: 1 in]
                  n517 = Less Or Equal?(x=w1486, y=w1483) -> (x <= y?=w1485:bool)
                  n518 = case shown="True" w1485 {
                    tunnel: [w1488 w1491] -> w1482
                    tunnel: w1487 -> [w1488 w1489]
                    frame False {
                    }
                    frame True {
                      n519 = Concatenate Strings("0" ("string"), w1489) -> (w1491:string)
                    }
                  }
                }
                frame 12 {
                  n520 = Index Array(array=w1494, index=w1496) -> (element=w1499:i32)
                  n521 = Number To Hexadecimal String(2:w1499) -> (0:w1500:string)  [unwired: 1 in]
                  n522 = Less Or Equal?(x=w1499, y=w1495) -> (x <= y?=w1498:bool)
                  n523 = case shown="True" w1498 {
                    tunnel: [w1501 w1504] -> w1497
                    tunnel: w1500 -> [w1501 w1502]
                    frame False {
                    }
                    frame True {
                      n524 = Concatenate Strings("0" ("string"), w1502) -> (w1504:string)
                    }
                  }
                  n525 = Concatenate Strings(w1493, w1497) -> (w1492:string)
                  n526 = Hexadecimal String To Number(string=w1492) -> ()  [unwired: 2 in, 2 out]
                }
                frame 13 {
                  n527 = Index Array(array=w1507, index=w1508) -> (element=w1510:i32)
                  n528 = Number To Hexadecimal String(2:w1510) -> (0:w1511:string)  [unwired: 1 in]
                  n529 = Less Or Equal?(x=w1510, y=w1505) -> (x <= y?=w1509:bool)
                  n530 = case shown="True" w1509 {
                    tunnel: [w1512 w1515] -> w1506
                    tunnel: w1511 -> [w1512 w1513]
                    frame False {
                    }
                    frame True {
                      n531 = Concatenate Strings("0" ("string"), w1513) -> (w1515:string)
                    }
                  }
                }
                frame 14 {
                  n532 = Index Array(array=w1518, index=w1520) -> (element=w1523:i32)
                  n533 = Number To Hexadecimal String(2:w1523) -> (0:w1524:string)  [unwired: 1 in]
                  n534 = Less Or Equal?(x=w1523, y=w1519) -> (x <= y?=w1522:bool)
                  n535 = case shown="True" w1522 {
                    tunnel: [w1525 w1528] -> w1521
                    tunnel: w1524 -> [w1525 w1526]
                    frame False {
                    }
                    frame True {
                      n536 = Concatenate Strings("0" ("string"), w1526) -> (w1528:string)
                    }
                  }
                  n537 = Concatenate Strings(w1517, w1521) -> (w1516:string)
                  n538 = Hexadecimal String To Number(string=w1516) -> ()  [unwired: 2 in, 2 out]
                }
                frame 15 {
                  n539 = Index Array(array=w1531, index=w1532) -> (element=w1534:i32)
                  n540 = Number To Hexadecimal String(2:w1534) -> (0:w1535:string)  [unwired: 1 in]
                  n541 = Less Or Equal?(x=w1534, y=w1530) -> (x <= y?=w1533:bool)
                  n542 = case shown="True" w1533 {
                    tunnel: [w1536 w1539] -> w1529
                    tunnel: w1535 -> [w1536 w1537]
                    frame False {
                    }
                    frame True {
                      n543 = Concatenate Strings("0" ("string"), w1537) -> (w1539:string)
                    }
                  }
                }
                frame 16 {
                  n544 = Index Array(array=w1542, index=w1544) -> (element=w1547:i32)
                  n545 = Number To Hexadecimal String(2:w1547) -> (0:w1548:string)  [unwired: 1 in]
                  n546 = Less Or Equal?(x=w1547, y=w1543) -> (x <= y?=w1546:bool)
                  n547 = case shown="True" w1546 {
                    tunnel: [w1549 w1552] -> w1545
                    tunnel: w1548 -> [w1549 w1550]
                    frame False {
                    }
                    frame True {
                      n548 = Concatenate Strings("0" ("string"), w1550) -> (w1552:string)
                    }
                  }
                  n549 = Concatenate Strings(w1541, w1545) -> (w1540:string)
                  n550 = Hexadecimal String To Number(string=w1540) -> ()  [unwired: 2 in, 2 out]
                }
                frame 17 {
                  n551 = Index Array(array=w1555, index=w1556) -> (element=w1558:i32)
                  n552 = Number To Hexadecimal String(2:w1558) -> (0:w1559:string)  [unwired: 1 in]
                  n553 = Less Or Equal?(x=w1558, y=w1554) -> (x <= y?=w1557:bool)
                  n554 = case shown="True" w1557 {
                    tunnel: [w1560 w1563] -> w1553
                    tunnel: w1559 -> [w1560 w1561]
                    frame False {
                    }
                    frame True {
                      n555 = Concatenate Strings("0" ("string"), w1561) -> (w1563:string)
                    }
                  }
                }
                frame 18 {
                  n556 = Index Array(array=w1567, index=w1568) -> (element=w1571:i32)
                  n557 = Number To Hexadecimal String(2:w1571) -> (0:w1572:string)  [unwired: 1 in]
                  n558 = Less Or Equal?(x=w1571, y=w1566) -> (x <= y?=w1570:bool)
                  n559 = case shown="True" w1570 {
                    tunnel: [w1573 w1576] -> w1569
                    tunnel: w1572 -> [w1573 w1574]
                    frame False {
                    }
                    frame True {
                      n560 = Concatenate Strings("0" ("string"), w1574) -> (w1576:string)
                    }
                  }
                  n561 = Concatenate Strings(w1565, w1569) -> (w1564:string)
                  n562 = Hexadecimal String To Number(string=w1564) -> ()  [unwired: 2 in, 2 out]
                }
                frame 19 {
                  n563 = Index Array(array=w1578, index=w1580) -> (element=w1582:i32)
                  n564 = Number To Hexadecimal String(2:w1582) -> (0:w1583:string)  [unwired: 1 in]
                  n565 = Less Or Equal?(x=w1582, y=w1579) -> (x <= y?=w1581:bool)
                  n566 = case shown="True" w1581 {
                    tunnel: [w1584 w1587] -> w1577
                    tunnel: w1583 -> [w1584 w1585]
                    frame False {
                    }
                    frame True {
                      n567 = Concatenate Strings("0" ("string"), w1585) -> (w1587:string)
                    }
                  }
                }
                frame 20 {
                  n568 = Index Array(array=w1592, index=w1593) -> (element=w1595:i32)
                  n569 = Number To Hexadecimal String(2:w1595) -> (0:w1596:string)  [unwired: 1 in]
                  n570 = Less Or Equal?(x=w1595, y=w1591) -> (x <= y?=w1594:bool)
                  n571 = case shown="True" w1594 {
                    tunnel: [w1597 w1600] -> w1590
                    tunnel: w1596 -> [w1597 w1598]
                    frame False {
                    }
                    frame True {
                      n572 = Concatenate Strings("0" ("string"), w1598) -> (w1600:string)
                    }
                  }
                  n573 = Concatenate Strings(w1589, w1590) -> (w1588:string)
                  n574 = Hexadecimal String To Number(string=w1588) -> ()  [unwired: 2 in, 2 out]
                }
                frame 21 {
                  n575 = Index Array(array=w1603, index=w1604) -> (element=w1606:i32)
                  n576 = Number To Hexadecimal String(2:w1606) -> (0:w1607:string)  [unwired: 1 in]
                  n577 = Less Or Equal?(x=w1606, y=w1602) -> (x <= y?=w1605:bool)
                  n578 = case shown="True" w1605 {
                    tunnel: [w1608 w1611] -> w1601
                    tunnel: w1607 -> [w1608 w1609]
                    frame False {
                    }
                    frame True {
                      n579 = Concatenate Strings("0" ("string"), w1609) -> (w1611:string)
                    }
                  }
                  n580 = Hexadecimal String To Number(string=w1601) -> ()  [unwired: 2 in, 2 out]
                }
                frame 22 {
                  n581 = Index Array(array=w1613, index=w1615) -> (element=w1617:i32)
                  n582 = Number To Hexadecimal String(2:w1617) -> (0:w1618:string)  [unwired: 1 in]
                  n583 = Less Or Equal?(x=w1617, y=w1614) -> (x <= y?=w1616:bool)
                  n584 = case shown="True" w1616 {
                    tunnel: [w1619 w1622] -> w1612
                    tunnel: w1618 -> [w1619 w1620]
                    frame False {
                    }
                    frame True {
                      n585 = Concatenate Strings("0" ("string"), w1620) -> (w1622:string)
                    }
                  }
                }
                frame 23 {
                  n586 = Index Array(array=w1626, index=w1627) -> (element=w1630:i32)
                  n587 = Number To Hexadecimal String(2:w1630) -> (0:w1631:string)  [unwired: 1 in]
                  n588 = Less Or Equal?(x=w1630, y=w1625) -> (x <= y?=w1629:bool)
                  n589 = case shown="True" w1629 {
                    tunnel: [w1632 w1635] -> w1628
                    tunnel: w1631 -> [w1632 w1633]
                    frame False {
                    }
                    frame True {
                      n590 = Concatenate Strings("0" ("string"), w1633) -> (w1635:string)
                    }
                  }
                  n591 = Concatenate Strings(w1623, w1628) -> (w1624:string)
                  n592 = Hexadecimal String To Number(string=w1624) -> ()  [unwired: 2 in, 2 out]
                }
                frame 24 {
                  n593 = Index Array(array=w1639, index=w1640) -> (element=w1643:i32)
                  n594 = Number To Hexadecimal String(2:w1643) -> (0:w1644:string)  [unwired: 1 in]
                  n595 = Less Or Equal?(x=w1643, y=w1638) -> (x <= y?=w1642:bool)
                  n596 = case shown="True" w1642 {
                    tunnel: [w1645 w1648] -> w1641
                    tunnel: w1644 -> [w1645 w1646]
                    frame False {
                    }
                    frame True {
                      n597 = Concatenate Strings("0" ("string"), w1646) -> (w1648:string)
                    }
                  }
                  n598 = Concatenate Strings(w1636, w1641) -> (w1637:string)
                }
                frame 25 {
                  n599 = Index Array(array=w1650, index=w1653) -> (element=w1656:i32)
                  n600 = Number To Hexadecimal String(2:w1656) -> (0:w1657:string)  [unwired: 1 in]
                  n601 = Less Or Equal?(x=w1656, y=w1651) -> (x <= y?=w1655:bool)
                  n602 = case shown="True" w1655 {
                    tunnel: [w1658 w1661] -> w1654
                    tunnel: w1657 -> [w1658 w1659]
                    frame False {
                    }
                    frame True {
                      n603 = Concatenate Strings("0" ("string"), w1659) -> (w1661:string)
                    }
                  }
                  n604 = Concatenate Strings(w1652, w1654) -> (w1649:string)
                  n605 = Hexadecimal String To Number(string=w1649) -> ()  [unwired: 2 in, 2 out]
                }
                frame 26 {
                  n606 = Index Array(array=w1664, index=w1665) -> (element=w1667:i32)
                  n607 = Number To Hexadecimal String(2:w1667) -> (0:w1668:string)  [unwired: 1 in]
                  n608 = Less Or Equal?(x=w1667, y=w1663) -> (x <= y?=w1666:bool)
                  n609 = case shown="True" w1666 {
                    tunnel: [w1669 w1672] -> w1662
                    tunnel: w1668 -> [w1669 w1670]
                    frame False {
                    }
                    frame True {
                      n610 = Concatenate Strings("0" ("string"), w1670) -> (w1672:string)
                    }
                  }
                }
                frame 27 {
                  n611 = Index Array(array=w1676, index=w1677) -> (element=w1680:i32)
                  n612 = Number To Hexadecimal String(2:w1680) -> (0:w1681:string)  [unwired: 1 in]
                  n613 = Less Or Equal?(x=w1680, y=w1673) -> (x <= y?=w1679:bool)
                  n614 = case shown="True" w1679 {
                    tunnel: [w1682 w1685] -> w1678
                    tunnel: w1681 -> [w1682 w1683]
                    frame False {
                    }
                    frame True {
                      n615 = Concatenate Strings("0" ("string"), w1683) -> (w1685:string)
                    }
                  }
                  n616 = Concatenate Strings(w1675, w1678) -> (w1674:string)
                }
                frame 28 {
                  n617 = Index Array(array=w1686, index=w1690) -> (element=w1693:i32)
                  n618 = Number To Hexadecimal String(2:w1693) -> (0:w1694:string)  [unwired: 1 in]
                  n619 = Less Or Equal?(x=w1693, y=w1689) -> (x <= y?=w1692:bool)
                  n620 = case shown="True" w1692 {
                    tunnel: [w1695 w1698] -> w1691
                    tunnel: w1694 -> [w1695 w1696]
                    frame False {
                    }
                    frame True {
                      n621 = Concatenate Strings("0" ("string"), w1696) -> (w1698:string)
                    }
                  }
                  n622 = Concatenate Strings(w1688, w1691) -> (w1687:string)
                }
                frame 29 {
                  n623 = Get Date/Time String() -> (date string=w1701:string, time string=w1699:string)  [unwired: 3 in]
                  n624 = Index Array(array=w1705, index=w1706) -> (element=w1709:i32)
                  n625 = Concatenate Strings(w1701, " a la(s)" ("string"), w1699) -> ()  [unwired: 1 out]
                  n626 = Number To Hexadecimal String(2:w1709) -> (0:w1710:string)  [unwired: 1 in]
                  n627 = Less Or Equal?(x=w1709, y=w1702) -> (x <= y?=w1708:bool)
                  n628 = case shown="True" w1708 {
                    tunnel: [w1711 w1714] -> w1707
                    tunnel: w1710 -> [w1711 w1712]
                    frame False {
                    }
                    frame True {
                      n629 = Concatenate Strings("0" ("string"), w1712) -> (w1714:string)
                    }
                  }
                  n630 = Concatenate Strings(w1704, w1707) -> (w1703:string)
                  n631 = Hexadecimal String To Number(string=w1703) -> ()  [unwired: 2 in, 2 out]
                }
              }
            }
          }
          frame "Monitor Set" {
          }
          frame "Schedule Set" {
            w1720 = "\t"
            w1723 = "\t"
            w1728 = "\r\n"
            n632 = property on="SCHEDULE SET" class="Clust (strict)"() -> ("Controls[]"=w1731:refnum<vi>[])  [unwired: 2 in, 2 out]
            n633 = property on="MONITOR SET" class="Clust (strict)"() -> ("Controls[]"=w1735:refnum<vi>[])  [unwired: 2 in, 2 out]
            n634 = for {
              N: 18 -> [_]
              tunnel: w1731 -> [w1756] mode=indexing
              shift-right: [w1752] -> w1729
              shift-left: "" -> [w1750]
              i -> [w1749]
              n635 = property class="Ctl"(reference=w1756) -> ("Value"=w1755:variant)  [unwired: 1 in, 2 out]
              n636 = Variant To Data(type=0.0 ("y"), Variant=w1755) -> (data=w1753:dbl)  [unwired: 1 in, 1 out]
              n637 = case shown="0, Default" w1749 {
                tunnel: w1753 -> [w1760 w1763 w1768 w1772 w1778 w1783 w1788 w1793 w1798 w1803 w1808 w1813 w1818 w1824 w1830 w1835 w1840 w1845]
                tunnel: [w1757 w1762 w1767 w1773 w1777 w1782 w1787 w1792 w1797 w1802 w1807 w1812 w1817 w1823 w1828 w1834 w1839 w1844] -> w1751
                frame 0, Default {
                  w1758 = "\t"
                  n638 = Number To Decimal String(number=w1760) -> (decimal integer string=w1759:string)  [unwired: 1 in]
                  n639 = Concatenate Strings("SQD", w1758, w1759, w1758) -> (w1757:string)
                }
                frame 1 {
                  w1764 = "\t"
                  n640 = Number To Decimal String(number=w1763) -> (decimal integer string=w1765:string)  [unwired: 1 in]
                  n641 = Concatenate Strings("SQZ", w1764, w1765, w1764) -> (w1762:string)
                }
                frame 2 {
                  w1769 = "\t"
                  n642 = Number To Decimal String(number=w1768) -> (decimal integer string=w1770:string)  [unwired: 1 in]
                  n643 = Concatenate Strings("UP1", w1769, w1770, w1769) -> (w1767:string)
                }
                frame 3 {
                  w1774 = "\t"
                  n644 = Number To Decimal String(number=w1772) -> (decimal integer string=w1775:string)  [unwired: 1 in]
                  n645 = Concatenate Strings("WELD1", w1774, w1775, w1774) -> (w1773:string)
                }
                frame 4 {
                  w1779 = "\t"
                  n646 = Number To Decimal String(number=w1778) -> (decimal integer string=w1780:string)  [unwired: 1 in]
                  n647 = Concatenate Strings("DOWN1", w1779, w1780, w1779) -> (w1777:string)
                }
                frame 5 {
                  w1784 = "\t"
                  n648 = Number To Decimal String(number=w1783) -> (decimal integer string=w1785:string)  [unwired: 1 in]
                  n649 = Concatenate Strings("COOL", w1784, w1785, w1784) -> (w1782:string)
                }
                frame 6 {
                  w1789 = "\t"
                  n650 = Number To Decimal String(number=w1788) -> (decimal integer string=w1790:string)  [unwired: 1 in]
                  n651 = Concatenate Strings("UP2", w1789, w1790, w1789) -> (w1787:string)
                }
                frame 7 {
                  w1794 = "\t"
                  n652 = Number To Decimal String(number=w1793) -> (decimal integer string=w1795:string)  [unwired: 1 in]
                  n653 = Concatenate Strings("WELD2", w1794, w1795, w1794) -> (w1792:string)
                }
                frame 8 {
                  w1799 = "\t"
                  n654 = Number To Decimal String(number=w1798) -> (decimal integer string=w1800:string)  [unwired: 1 in]
                  n655 = Concatenate Strings("DOWN2", w1799, w1800, w1799) -> (w1797:string)
                }
                frame 9 {
                  w1804 = "\t"
                  n656 = Number To Decimal String(number=w1803) -> (decimal integer string=w1805:string)  [unwired: 1 in]
                  n657 = Concatenate Strings("HOLD", w1804, w1805, w1804) -> (w1802:string)
                }
                frame 10 {
                  w1809 = "\t"
                  n658 = Number To Decimal String(number=w1808) -> (decimal integer string=w1810:string)  [unwired: 1 in]
                  n659 = Concatenate Strings("OFF", w1809, w1810, w1809) -> (w1807:string)
                }
                frame 11 {
                  w1814 = "\t"
                  n660 = Number To Decimal String(number=w1813) -> (decimal integer string=w1815:string)  [unwired: 1 in]
                  n661 = Concatenate Strings("%HEAT1", w1814, w1815, w1814) -> (w1812:string)
                }
                frame 12 {
                  w1819 = "\t"
                  n662 = Number To Decimal String(number=w1818) -> (decimal integer string=w1820:string)  [unwired: 1 in]
                  n663 = Concatenate Strings("%HEAT2", w1819, w1820, w1819) -> (w1817:string)
                }
                frame 13 {
                  w1825 = "\t"
                  n664 = Number To Fractional String(number=w1824, precision (6)=i16 2) -> (F-format string=w1826:string)  [unwired: 2 in]
                  n665 = Concatenate Strings("CURRENT1", w1825, w1826, w1825) -> (w1823:string)
                }
                frame 14 {
                  w1831 = "\t"
                  n666 = Number To Fractional String(number=w1830, precision (6)=i16 2) -> (F-format string=w1832:string)  [unwired: 2 in]
                  n667 = Concatenate Strings("CURRENT2", w1831, w1832, w1831) -> (w1828:string)
                }
                frame 15 {
                  w1836 = "\t"
                  n668 = Number To Decimal String(number=w1835) -> (decimal integer string=w1837:string)  [unwired: 1 in]
                  n669 = Concatenate Strings("IMPULSE", w1836, w1837, w1836) -> (w1834:string)
                }
                frame 16 {
                  w1841 = "\t"
                  n670 = Number To Decimal String(number=w1840) -> (decimal integer string=w1842:string)  [unwired: 1 in]
                  n671 = Concatenate Strings("FORCE", w1841, w1842, w1841) -> (w1839:string)
                }
                frame 17 {
                  w1846 = "\t"
                  n672 = Number To Decimal String(number=w1845) -> (decimal integer string=w1847:string)  [unwired: 1 in]
                  n673 = Concatenate Strings("FORCE CHANNEL", w1846, w1847, w1846) -> (w1844:string)
                }
              }
              n674 = Concatenate Strings(w1750, w1751) -> (w1752:string)
            }
            n675 = for {
              N: 16 -> [_]
              tunnel: w1735 -> [w1856] mode=indexing
              shift-right: [w1851] -> w1733
              shift-left: "" -> [w1850]
              i -> [w1853]
              n676 = property class="Ctl"(reference=w1856) -> ("Value"=w1855:variant)  [unwired: 1 in, 2 out]
              n677 = Variant To Data(type=0.0 ("y"), Variant=w1855) -> (data=w1852:dbl)  [unwired: 1 in, 1 out]
              n678 = case shown="8" w1853 {
                tunnel: w1852 -> [w1860 w1863 w1868 w1872 w1878 w1883 w1888 w1893 w1898 w1903 w1908 w1914 w1920 w1925 w1931 w1936]
                tunnel: [w1857 w1862 w1867 w1873 w1877 w1882 w1887 w1892 w1897 w1902 w1907 w1912 w1918 w1924 w1929 w1935] -> w1849
                frame 0, Default {
                  w1858 = "\t"
                  n679 = Number To Decimal String(number=w1860) -> (decimal integer string=w1859:string)  [unwired: 1 in]
                  n680 = Concatenate Strings("HIGH1C", w1858, w1859, w1858) -> (w1857:string)
                }
                frame 1 {
                  w1864 = "\t"
                  n681 = Number To Decimal String(number=w1863) -> (decimal integer string=w1865:string)  [unwired: 1 in]
                  n682 = Concatenate Strings("LOW1C", w1864, w1865, w1864) -> (w1862:string)
                }
                frame 2 {
                  w1869 = "\t"
                  n683 = Number To Decimal String(number=w1868) -> (decimal integer string=w1870:string)  [unwired: 1 in]
                  n684 = Concatenate Strings("HIGH2C", w1869, w1870, w1869) -> (w1867:string)
                }
                frame 3 {
                  w1874 = "\t"
                  n685 = Number To Decimal String(number=w1872) -> (decimal integer string=w1875:string)  [unwired: 1 in]
                  n686 = Concatenate Strings("LOW2C", w1874, w1875, w1874) -> (w1873:string)
                }
                frame 4 {
                  w1879 = "\t"
                  n687 = Number To Decimal String(number=w1878) -> (decimal integer string=w1880:string)  [unwired: 1 in]
                  n688 = Concatenate Strings("ANGLE1", w1879, w1880, w1879) -> (w1877:string)
                }
                frame 5 {
                  w1884 = "\t"
                  n689 = Number To Decimal String(number=w1883) -> (decimal integer string=w1885:string)  [unwired: 1 in]
                  n690 = Concatenate Strings("ANGLE2", w1884, w1885, w1884) -> (w1882:string)
                }
                frame 6 {
                  w1889 = "\t"
                  n691 = Number To Decimal String(number=w1888) -> (decimal integer string=w1890:string)  [unwired: 1 in]
                  n692 = Concatenate Strings("LIMIT", w1889, w1890, w1889) -> (w1887:string)
                }
                frame 7 {
                  w1894 = "\t"
                  n693 = Number To Decimal String(number=w1893) -> (decimal integer string=w1895:string)  [unwired: 1 in]
                  n694 = Concatenate Strings("START", w1894, w1895, w1894) -> (w1892:string)
                }
                frame 8 {
                  w1899 = "\t"
                  n695 = Number To Decimal String(number=w1898) -> (decimal integer string=w1900:string)  [unwired: 1 in]
                  n696 = Concatenate Strings("WELD MODE", w1899, w1900, w1899) -> (w1897:string)
                }
                frame 9 {
                  w1904 = "\t"
                  n697 = Number To Decimal String(number=w1903) -> (decimal integer string=w1905:string)  [unwired: 1 in]
                  n698 = Concatenate Strings("LOP", w1904, w1905, w1904) -> (w1902:string)
                }
                frame 10 {
                  w1909 = "\t"
                  n699 = Number To Decimal String(number=w1908) -> (decimal integer string=w1910:string)  [unwired: 1 in]
                  n700 = Concatenate Strings("HIP", w1909, w1910, w1909) -> (w1907:string)
                }
                frame 11 {
                  w1915 = "\t"
                  n701 = Number To Fractional String(number=w1914, precision (6)=i16 2) -> (F-format string=w1916:string)  [unwired: 2 in]
                  n702 = Concatenate Strings("VOLTHIW1", w1915, w1916, w1915) -> (w1912:string)
                }
                frame 12 {
                  w1921 = "\t"
                  n703 = Number To Fractional String(number=w1920, precision (6)=i16 2) -> (F-format string=w1922:string)  [unwired: 2 in]
                  n704 = Concatenate Strings("VOLTLOW1", w1921, w1922, w1921) -> (w1918:string)
                }
                frame 13 {
                  w1926 = "\t"
                  n705 = Number To Fractional String(number=w1925) -> (F-format string=w1927:string)  [unwired: 3 in]
                  n706 = Concatenate Strings("VOLTHIW2", w1926, w1927, w1926) -> (w1924:string)
                }
                frame 14 {
                  w1932 = "\t"
                  n707 = Number To Fractional String(number=w1931, precision (6)=i16 2) -> (F-format string=w1933:string)  [unwired: 2 in]
                  n708 = Concatenate Strings("VOLTLOW2", w1932, w1933, w1932) -> (w1929:string)
                }
                frame 15 {
                  w1937 = "\t"
                  n709 = Number To Decimal String(number=w1936) -> (decimal integer string=w1938:string)  [unwired: 1 in]
                  n710 = Concatenate Strings("FIRE", w1937, w1938, w1937) -> (w1935:string)
                }
              }
              n711 = Concatenate Strings(w1850, w1849) -> (w1851:string)
            }
            n712 = local read "SCHEDULE"() -> (w1724:u32)
            n713 = Number To Decimal String(number=w1724) -> (decimal integer string=w1725:string)  [unwired: 1 in]
            n714 = Concatenate Strings("SCHEDULE", w1723, w1725, w1723) -> (w1719:string)
            n715 = call <vilib>:"Application Directory.vi"() -> ("Application Directory"=w1747:path)
            n716 = Build Path(base path=w1747, name or relative path="schedules.txt") -> (appended path=w1748:path)
            n717 = Get Date/Time String() -> (date string=w1722:string, time string=w1721:string)  [unwired: 3 in]
            n718 = Open/Create/Replace File(file path (use dialog)=w1748) -> (refnum out=w1740:refnum<file>, error out=w1741:errorcluster)  [unwired: 5 in, 1 out]
            n719 = Get File Size(file=w1740, error in=w1741) -> (refnum out=w1739:refnum<file>, size (in bytes)=w1738:i64, 0:w1742:errorcluster)
            n720 = Concatenate Strings(w1722, w1720, w1721, w1720, w1719, w1733, w1728, w1729, w1728, w1728) -> (w1727:string)
            n721 = Set File Position(offset (in bytes) (0)=w1738, refnum=w1739, error in=w1742) -> (refnum out=w1737:refnum<file>, error out=w1743:errorcluster)  [unwired: 1 in]
            n722 = Write to Text File(file (use dialog)=w1737, text=w1727, error in=w1743) -> (refnum out=w1745:refnum<file>, error out=w1744:errorcluster)  [unwired: 1 in, 1 out]
            n723 = Close File(refnum=w1745, error in=w1744) -> ()  [unwired: 2 out]
          }
          frame "ACK" {
          }
          frame "Remote" {
          }
        }
        n724 = Or(x=w741, y=w742) -> (x .or. y?=w740:i32)
        n725 = case shown="1, Default" w740 {
          tunnel: [FGV_Machine_states."Idle" ("Estado") FGV_Machine_states."Wait" ("Estado")] -> w744
          frame 0 {
          }
          frame 1, Default {
          }
        }
        n726 = Bundle By Name(cluster=w746, "State"=w744, "Status?"=w739, "Case"=w738) -> (w745:T2)
      }
      frame "Stop" {
        n727 = Bundle By Name(cluster=w1946, "stopVI"=TRUE) -> (w1945:T2)
      }
    }
    "OK" <- w6
    n728 = Unbundle By Name(w5) -> ("stopVI"=w4:bool)
  }
